vi "auto foil kinematics kl v4.1 08 01 2016.vi"() -> ()   [LabVIEW 2013]
uses:
  <vilib>/Utility/file.llb/Write To Spreadsheet File (DBL).vi
  <vilib>/Utility/file.llb/Write To Spreadsheet File (string).vi
  <vilib>/vision/NI_Vision_Development_Module.lvlib
panel:
  in  "X coordinate \nwithin gap\n(in pixels)":dbl=550.0
  in  "ON for 2 foil\nsegments":bool
  in  "Start frame":i32=1
  in  "ON to \nsimulate rod":bool
  in  "ON for pitch,\nOFF if NO pitch":bool=TRUE
  in  "Rod width (mm)":dbl=10.0
  out "Rotated/Mirrored image":T1(plugin-control)
  in  "Frame increment\nfor kinematics avi":i32=20
  in  "Flip along\nhorizontal line":bool
  in  "Flip along\nvertical line":bool
  in  "Save amps of\noscillation\nto txt file":bool
  in  "Save splines\nfor snapshot\ngeneration":bool
  in  "File path for snapshot splines (dialog if empty)":path=path "C:/Users/Lauder Lab/Desktop/snapshotstest.txt"
  in  "Number of\ncycles":i32=2
  in  "Foil chord (m)":dbl=0.18
  in  "File path for amplitudes of oscillation (dialog if empty)":path=path "C:/Users/Lauder Lab/Desktop/testcol.txt"
  in  "Increment for\nsaving extra\n splines":i32=20
  in  "File path for extra kinematics splines (dialog if empty)":path=path "C:/Users/Lauder Lab/Desktop/splinestest.txt"
  in  "For raw detected\nsurface:\nOn for mm,\nOff for pixels":bool
  in  "Save raw \ndetected\nsurface to\nspreadsheet":bool
  in  "File path for surfaces (dialog if empty)":path=path "C:/Users/Lauder Lab/Desktop/test.txt"
  in  "Save extra splines\n(at increment)\nto txt file":bool
  in  "Save an avi\nanimation":bool
  in  "File path for kinematics avi":path=path "C:/Users/Lauder Lab/Desktop/movie.avi"
  in  "Rotate\n90 deg (CCW)":bool
  in  "Rotate\n180 deg":bool
  in  "On for\ntest display":bool=TRUE
  in  "Number of frames\nto analyze":i32=1000
  out "surface":cluster{i32, "Rows":i32}[](graph)=[{0, "Rows"=0}, {1, "Rows"=0}, {2, "Rows"=0}, {3, "Rows"=0}, {4, "Rows"=0}, {5, "Rows"=0}, {6, "Rows"=0}, {7, "Rows"=0}, {8, "Rows"=0}, {9, "Rows"=0}, {10, "Rows"=0}, {11, "Rows"=0}, {12, "Rows"=0}, {13, "Rows"=0}, {14, "Rows"=0}, {15, "Rows"=0}, {16, "Rows"=0}, {17, "Rows"=0}, {18, "Rows"=0}, {19, "Rows"=0}, {20, "Rows"=0}, {21, "Rows"=0}, {22, "Rows"=0}, {23, "Rows"=0}, {24, "Rows"=0}, {25, "Rows"=0}, {26, "Rows"=0}, {27, "Rows"=0}, {28, "Rows"=0}, {29, "Rows"=0}, {30, "Rows"=0}, {31, "Rows"=0}, {32, "Rows"=0}, {33, "Rows"=0}, {34, "Rows"=0}, {35, "Rows"=0}, {36, "Rows"=0}, {37, "Rows"=0}, {38, "Rows"=0}, {39, "Rows"=0}, {40, "Rows"=0}, {41, "Rows"=0}, {42, "Rows"=0}, {43, "Rows"=0}, {44, "Rows"=0}, {45, "Rows"=0}, {46, "Rows"=0}, {47, "Rows"=0}, {48, "Rows"=0}, {49, "Rows"=0}, {50, "Rows"=0}, {51, "Rows"=0}, {52, "Rows"=0}, {53, "Rows"=0}, {54, "Rows"=0}, {55, "Rows"=0}, {56, "Rows"=0}, {57, "Rows"=0}, {58, "Rows"=0}, {59, "Rows"=0}, {60, "Rows"=0}, {61, "Rows"=0}, {62, "Rows"=0}, {63, "Rows"=0}, {64, "Rows"=0}, {65, "Rows"=0}, {66, "Rows"=0}, {67, "Rows"=0}, {68, "Rows"=0}, {69, "Rows"=0}, {70, "Rows"=0}, {71, "Rows"=0}, {72, "Rows"=0}, {73, "Rows"=0}, {74, "Rows"=0}, {75, "Rows"=0}, {76, "Rows"=0}, {77, "Rows"=0}, {78, "Rows"=0}, {79, "Rows"=0}, {80, "Rows"=0}, {81, "Rows"=0}, {82, "Rows"=0}, {83, "Rows"=0}, {84, "Rows"=0}, {85, "Rows"=0}, {86, "Rows"=0}, {87, "Rows"=0}, {88, "Rows"=0}, {89, "Rows"=0}, {90, "Rows"=0}, {91, "Rows"=0}, {92, "Rows"=0}, {93, "Rows"=0}, {94, "Rows"=0}, {95, "Rows"=0}, {96, "Rows"=0}, {97, "Rows"=0}, {98, "Rows"=0}, {99, "Rows"=0}, {100, "Rows"=0}, {101, "Rows"=0}, {102, "Rows"=0}, {103, "Rows"=0}, {104, "Rows"=0}, {105, "Rows"=0}, {106, "Rows"=0}, {107, "Rows"=0}, {108, "Rows"=0}, {109, "Rows"=0}, {110, "Rows"=0}, {111, "Rows"=0}, {112, "Rows"=0}, {113, "Rows"=0}, {114, "Rows"=0}, {115, "Rows"=0}, {116, "Rows"=0}, {117, "Rows"=0}, {118, "Rows"=0}, {119, "Rows"=0}, {120, "Rows"=0}, {121, "Rows"=0}, {122, "Rows"=0}, {123, "Rows"=0}, {124, "Rows"=0}, {125, "Rows"=0}, {126, "Rows"=0}, {127, "Rows"=0}, {128, "Rows"=0}, {129, "Rows"=0}, {130, "Rows"=0}, {131, "Rows"=0}, {132, "Rows"=0}, {133, "Rows"=0}, {134, "Rows"=0}, {135, "Rows"=0}, {136, "Rows"=0}, {137, "Rows"=0}, {138, "Rows"=0}, {139, "Rows"=0}, {140, "Rows"=0}, {141, "Rows"=0}, {142, "Rows"=0}, {143, "Rows"=0}, {144, "Rows"=0}, {145, "Rows"=0}, {146, "Rows"=0}, {147, "Rows"=0}, {148, "Rows"=0}, {149, "Rows"=0}, {150, "Rows"=0}, {151, "Rows"=0}, {152, "Rows"=0}, {153, "Rows"=0}, {154, "Rows"=0}, {155, "Rows"=0}, {156, "Rows"=0}, {157, "Rows"=0}, {158, "Rows"=0}, {159, "Rows"=0}, {160, "Rows"=0}, {161, "Rows"=0}, {162, "Rows"=0}, {163, "Rows"=0}, {164, "Rows"=0}, {165, "Rows"=0}, {166, "Rows"=0}, {167, "Rows"=0}, {168, "Rows"=0}, {169, "Rows"=0}, {170, "Rows"=0}, {171, "Rows"=0}, {172, "Rows"=0}, {173, "Rows"=0}, {174, "Rows"=0}, {175, "Rows"=0}, {176, "Rows"=0}, {177, "Rows"=0}, {178, "Rows"=0}, {179, "Rows"=0}, {180, "Rows"=0}, {181, "Rows"=0}, {182, "Rows"=0}, {183, "Rows"=0}, {184, "Rows"=0}, {185, "Rows"=0}, {186, "Rows"=0}, {187, "Rows"=0}, {188, "Rows"=0}, {189, "Rows"=0}, {190, "Rows"=0}, {191, "Rows"=0}, {192, "Rows"=0}, {193, "Rows"=0}, {194, "Rows"=0}, {195, "Rows"=0}, {196, "Rows"=0}, {197, "Rows"=0}, {198, "Rows"=0}, {199, "Rows"=0}, {200, "Rows"=0}, {201, "Rows"=0}, {202, "Rows"=0}, {203, "Rows"=0}, {204, "Rows"=0}, {205, "Rows"=0}, {206, "Rows"=0}, {207, "Rows"=0}, {208, "Rows"=0}, {209, "Rows"=0}, {210, "Rows"=0}, {211, "Rows"=0}, {212, "Rows"=0}, {213, "Rows"=0}, {214, "Rows"=0}, {215, "Rows"=0}, {216, "Rows"=0}, {217, "Rows"=0}, {218, "Rows"=0}, {219, "Rows"=0}, {220, "Rows"=0}, {221, "Rows"=0}, {222, "Rows"=0}, {223, "Rows"=0}, {224, "Rows"=0}, {225, "Rows"=582}, {226, "Rows"=582}, {227, "Rows"=581}, {228, "Rows"=580}, {229, "Rows"=579}, {230, "Rows"=579}, {231, "Rows"=579}, {232, "Rows"=579}, {233, "Rows"=579}, {234, "Rows"=579}, {235, "Rows"=579}, {236, "Rows"=579}, {237, "Rows"=579}, {238, "Rows"=579}, {239, "Rows"=579}, {240, "Rows"=579}, {241, "Rows"=579}, {242, "Rows"=578}, {243, "Rows"=578}, {244, "Rows"=578}, {245, "Rows"=578}, {246, "Rows"=578}, {247, "Rows"=578}, {248, "Rows"=578}, {249, "Rows"=578}, {250, "Rows"=578}, {251, "Rows"=578}, {252, "Rows"=578}, {253, "Rows"=578}, {254, "Rows"=578}, {255, "Rows"=578}, {256, "Rows"=578}, {257, "Rows"=578}, {258, "Rows"=577}, {259, "Rows"=577}, {260, "Rows"=577}, {261, "Rows"=577}, {262, "Rows"=577}, {263, "Rows"=577}, {264, "Rows"=577}, {265, "Rows"=577}, {266, "Rows"=577}, {267, "Rows"=577}, {268, "Rows"=577}, {269, "Rows"=577}, {270, "Rows"=577}, {271, "Rows"=577}, {272, "Rows"=577}, {273, "Rows"=577}, {274, "Rows"=577}, {275, "Rows"=577}, {276, "Rows"=576}, {277, "Rows"=576}, {278, "Rows"=576}, {279, "Rows"=576}, {280, "Rows"=576}, {281, "Rows"=576}, {282, "Rows"=576}, {283, "Rows"=576}, {284, "Rows"=576}, {285, "Rows"=576}, {286, "Rows"=576}, {287, "Rows"=576}, {288, "Rows"=576}, {289, "Rows"=576}, {290, "Rows"=576}, {291, "Rows"=576}, {292, "Rows"=576}, {293, "Rows"=575}, {294, "Rows"=575}, {295, "Rows"=575}, {296, "Rows"=575}, {297, "Rows"=575}, {298, "Rows"=575}, {299, "Rows"=575}, {300, "Rows"=575}, {301, "Rows"=575}, {302, "Rows"=574}, {303, "Rows"=574}, {304, "Rows"=574}, {305, "Rows"=574}, {306, "Rows"=574}, {307, "Rows"=574}, {308, "Rows"=574}, {309, "Rows"=574}, {310, "Rows"=574}, {311, "Rows"=574}, {312, "Rows"=574}, {313, "Rows"=574}, {314, "Rows"=573}, {315, "Rows"=573}, {316, "Rows"=573}, {317, "Rows"=573}, {318, "Rows"=573}, {319, "Rows"=573}, {320, "Rows"=573}, {321, "Rows"=573}, {322, "Rows"=573}, {323, "Rows"=573}, {324, "Rows"=572}, {325, "Rows"=572}, {326, "Rows"=572}, {327, "Rows"=572}, {328, "Rows"=572}, {329, "Rows"=572}, {330, "Rows"=572}, {331, "Rows"=572}, {332, "Rows"=571}, {333, "Rows"=572}, {334, "Rows"=571}, {335, "Rows"=571}, {336, "Rows"=571}, {337, "Rows"=571}, {338, "Rows"=570}, {339, "Rows"=571}, {340, "Rows"=571}, {341, "Rows"=570}, {342, "Rows"=570}, {343, "Rows"=570}, {344, "Rows"=570}, {345, "Rows"=570}, {346, "Rows"=570}, {347, "Rows"=570}, {348, "Rows"=569}, {349, "Rows"=569}, {350, "Rows"=569}, {351, "Rows"=569}, {352, "Rows"=569}, {353, "Rows"=569}, {354, "Rows"=569}, {355, "Rows"=569}, {356, "Rows"=568}, {357, "Rows"=568}, {358, "Rows"=568}, {359, "Rows"=568}, {360, "Rows"=568}, {361, "Rows"=568}, {362, "Rows"=567}, {363, "Rows"=567}, {364, "Rows"=567}, {365, "Rows"=567}, {366, "Rows"=567}, {367, "Rows"=566}, {368, "Rows"=566}, {369, "Rows"=566}, {370, "Rows"=566}, {371, "Rows"=566}, {372, "Rows"=566}, {373, "Rows"=565}, {374, "Rows"=565}, {375, "Rows"=565}, {376, "Rows"=565}, {377, "Rows"=565}, {378, "Rows"=565}, {379, "Rows"=564}, {380, "Rows"=564}, {381, "Rows"=564}, {382, "Rows"=564}, {383, "Rows"=564}, {384, "Rows"=564}, {385, "Rows"=564}, {386, "Rows"=563}, {387, "Rows"=563}, {388, "Rows"=563}, {389, "Rows"=563}, {390, "Rows"=562}, {391, "Rows"=562}, {392, "Rows"=562}, {393, "Rows"=562}, {394, "Rows"=562}, {395, "Rows"=562}, {396, "Rows"=562}, {397, "Rows"=561}, {398, "Rows"=561}, {399, "Rows"=561}, {400, "Rows"=561}, {401, "Rows"=561}, {402, "Rows"=560}, {403, "Rows"=560}, {404, "Rows"=560}, {405, "Rows"=560}, {406, "Rows"=560}, {407, "Rows"=560}, {408, "Rows"=560}, {409, "Rows"=559}, {410, "Rows"=559}, {411, "Rows"=559}, {412, "Rows"=559}, {413, "Rows"=558}, {414, "Rows"=558}, {415, "Rows"=558}, {416, "Rows"=558}, {417, "Rows"=558}, {418, "Rows"=557}, {419, "Rows"=557}, {420, "Rows"=557}, {421, "Rows"=557}, {422, "Rows"=557}, {423, "Rows"=557}, {424, "Rows"=556}, {425, "Rows"=556}, {426, "Rows"=556}, {427, "Rows"=556}, {428, "Rows"=556}, {429, "Rows"=555}, {430, "Rows"=555}, {431, "Rows"=555}, {432, "Rows"=555}, {433, "Rows"=554}, {434, "Rows"=554}, {435, "Rows"=554}, {436, "Rows"=554}, {437, "Rows"=554}, {438, "Rows"=554}, {439, "Rows"=553}, {440, "Rows"=553}, {441, "Rows"=553}, {442, "Rows"=553}, {443, "Rows"=553}, {444, "Rows"=553}, {445, "Rows"=552}, {446, "Rows"=552}, {447, "Rows"=552}, {448, "Rows"=552}, {449, "Rows"=552}, {450, "Rows"=551}, {451, "Rows"=551}, {452, "Rows"=551}, {453, "Rows"=551}, {454, "Rows"=550}, {455, "Rows"=550}, {456, "Rows"=550}, {457, "Rows"=550}, {458, "Rows"=550}, {459, "Rows"=549}, {460, "Rows"=549}, {461, "Rows"=549}, {462, "Rows"=549}, {463, "Rows"=549}, {464, "Rows"=548}, {465, "Rows"=548}, {466, "Rows"=548}, {467, "Rows"=548}, {468, "Rows"=548}, {469, "Rows"=548}, {470, "Rows"=547}, {471, "Rows"=547}, {472, "Rows"=547}, {473, "Rows"=547}, {474, "Rows"=547}, {475, "Rows"=546}, {476, "Rows"=546}, {477, "Rows"=546}, {478, "Rows"=546}, {479, "Rows"=546}, {480, "Rows"=546}, {481, "Rows"=546}, {482, "Rows"=545}, {483, "Rows"=545}, {484, "Rows"=545}, {485, "Rows"=545}, {486, "Rows"=544}, {487, "Rows"=544}, {488, "Rows"=544}, {489, "Rows"=544}, {490, "Rows"=544}, {491, "Rows"=541}, {492, "Rows"=541}, {493, "Rows"=543}, {494, "Rows"=543}, {495, "Rows"=542}, {496, "Rows"=542}, {497, "Rows"=542}, {498, "Rows"=542}, {499, "Rows"=541}, {500, "Rows"=541}, {501, "Rows"=541}, {502, "Rows"=541}, {503, "Rows"=541}, {504, "Rows"=541}, {505, "Rows"=540}, {506, "Rows"=540}, {507, "Rows"=540}, {508, "Rows"=540}, {509, "Rows"=540}, {510, "Rows"=539}, {511, "Rows"=539}, {512, "Rows"=539}, {513, "Rows"=539}, {514, "Rows"=539}, {515, "Rows"=538}, {516, "Rows"=538}, {517, "Rows"=538}, {518, "Rows"=537}, {519, "Rows"=537}, {520, "Rows"=537}, {521, "Rows"=537}, {522, "Rows"=537}, {523, "Rows"=536}, {524, "Rows"=536}, {525, "Rows"=536}, {526, "Rows"=536}, {527, "Rows"=536}, {528, "Rows"=535}, {529, "Rows"=535}, {530, "Rows"=535}, {531, "Rows"=535}, {532, "Rows"=535}, {533, "Rows"=534}, {534, "Rows"=534}, {535, "Rows"=534}, {536, "Rows"=534}, {537, "Rows"=534}, {538, "Rows"=533}, {539, "Rows"=533}, {540, "Rows"=533}, {541, "Rows"=533}, {542, "Rows"=533}, {543, "Rows"=532}, {544, "Rows"=532}, {545, "Rows"=532}, {546, "Rows"=532}, {547, "Rows"=532}, {548, "Rows"=531}, {549, "Rows"=531}, {550, "Rows"=531}, {551, "Rows"=531}, {552, "Rows"=531}, {553, "Rows"=530}, {554, "Rows"=530}, {555, "Rows"=530}, {556, "Rows"=530}, {557, "Rows"=530}, {558, "Rows"=530}, {559, "Rows"=529}, {560, "Rows"=529}, {561, "Rows"=529}, {562, "Rows"=529}, {563, "Rows"=528}, {564, "Rows"=528}, {565, "Rows"=528}, {566, "Rows"=528}, {567, "Rows"=527}, {568, "Rows"=527}, {569, "Rows"=527}, {570, "Rows"=527}, {571, "Rows"=526}, {572, "Rows"=526}, {573, "Rows"=526}, {574, "Rows"=526}, {575, "Rows"=526}, {576, "Rows"=526}, {577, "Rows"=525}, {578, "Rows"=525}, {579, "Rows"=525}, {580, "Rows"=524}, {581, "Rows"=524}, {582, "Rows"=524}, {583, "Rows"=524}, {584, "Rows"=524}, {585, "Rows"=524}, {586, "Rows"=524}, {587, "Rows"=523}, {588, "Rows"=523}, {589, "Rows"=523}, {590, "Rows"=523}, {591, "Rows"=522}, {592, "Rows"=522}, {593, "Rows"=522}, {594, "Rows"=522}, {595, "Rows"=520}, {596, "Rows"=521}, {597, "Rows"=521}, {598, "Rows"=521}, {599, "Rows"=520}, {600, "Rows"=520}, {601, "Rows"=520}, {602, "Rows"=520}, {603, "Rows"=519}, {604, "Rows"=519}, {605, "Rows"=519}, {606, "Rows"=519}, {607, "Rows"=518}, {608, "Rows"=518}, {609, "Rows"=517}, {610, "Rows"=517}, {611, "Rows"=517}, {612, "Rows"=516}, {613, "Rows"=516}, {614, "Rows"=516}, {615, "Rows"=516}, {616, "Rows"=516}, {617, "Rows"=516}, {618, "Rows"=516}, {619, "Rows"=516}, {620, "Rows"=516}, {621, "Rows"=516}, {622, "Rows"=516}, {623, "Rows"=516}, {624, "Rows"=515}, {625, "Rows"=514}, {626, "Rows"=513}, {627, "Rows"=513}, {628, "Rows"=513}, {629, "Rows"=513}, {630, "Rows"=513}, {631, "Rows"=512}, {632, "Rows"=512}, {633, "Rows"=511}, {634, "Rows"=511}, {635, "Rows"=511}, {636, "Rows"=511}, {637, "Rows"=511}, {638, "Rows"=510}, {639, "Rows"=510}, {640, "Rows"=509}, {641, "Rows"=508}, {642, "Rows"=508}, {643, "Rows"=507}, {644, "Rows"=507}, {645, "Rows"=507}, {646, "Rows"=506}, {647, "Rows"=506}, {648, "Rows"=505}, {649, "Rows"=505}, {650, "Rows"=504}, {651, "Rows"=504}, {652, "Rows"=504}, {653, "Rows"=503}, {654, "Rows"=502}, {655, "Rows"=501}, {656, "Rows"=501}, {657, "Rows"=501}, {658, "Rows"=500}, {659, "Rows"=499}, {660, "Rows"=498}, {661, "Rows"=498}, {662, "Rows"=498}, {663, "Rows"=498}, {664, "Rows"=497}, {665, "Rows"=496}, {666, "Rows"=496}, {667, "Rows"=495}, {668, "Rows"=494}, {669, "Rows"=494}, {670, "Rows"=493}, {671, "Rows"=493}, {672, "Rows"=492}, {673, "Rows"=491}, {674, "Rows"=491}, {675, "Rows"=490}, {676, "Rows"=489}, {677, "Rows"=489}, {678, "Rows"=488}, {679, "Rows"=488}, {680, "Rows"=487}, {681, "Rows"=486}, {682, "Rows"=486}, {683, "Rows"=485}, {684, "Rows"=484}, {685, "Rows"=483}, {686, "Rows"=483}, {687, "Rows"=482}, {688, "Rows"=481}, {689, "Rows"=480}, {690, "Rows"=479}, {691, "Rows"=479}, {692, "Rows"=478}, {693, "Rows"=478}, {694, "Rows"=477}, {695, "Rows"=476}, {696, "Rows"=476}, {697, "Rows"=475}, {698, "Rows"=474}, {699, "Rows"=473}, {700, "Rows"=472}, {701, "Rows"=472}, {702, "Rows"=471}, {703, "Rows"=470}, {704, "Rows"=470}, {705, "Rows"=469}, {706, "Rows"=468}, {707, "Rows"=467}, {708, "Rows"=467}, {709, "Rows"=466}, {710, "Rows"=464}, {711, "Rows"=463}, {712, "Rows"=463}, {713, "Rows"=463}, {714, "Rows"=462}, {715, "Rows"=461}, {716, "Rows"=460}, {717, "Rows"=459}, {718, "Rows"=458}, {719, "Rows"=458}, {720, "Rows"=457}, {721, "Rows"=456}, {722, "Rows"=455}, {723, "Rows"=455}, {724, "Rows"=454}, {725, "Rows"=453}, {726, "Rows"=452}, {727, "Rows"=451}, {728, "Rows"=450}, {729, "Rows"=450}, {730, "Rows"=449}, {731, "Rows"=448}, {732, "Rows"=447}, {733, "Rows"=447}, {734, "Rows"=446}, {735, "Rows"=445}, {736, "Rows"=444}, {737, "Rows"=443}, {738, "Rows"=442}, {739, "Rows"=441}, {740, "Rows"=440}, {741, "Rows"=439}, {742, "Rows"=438}, {743, "Rows"=438}, {744, "Rows"=437}, {745, "Rows"=436}, {746, "Rows"=436}, {747, "Rows"=435}, {748, "Rows"=434}, {749, "Rows"=433}, {750, "Rows"=432}, {751, "Rows"=432}, {752, "Rows"=431}, {753, "Rows"=430}, {754, "Rows"=429}, {755, "Rows"=428}, {756, "Rows"=427}, {757, "Rows"=426}, {758, "Rows"=425}, {759, "Rows"=425}, {760, "Rows"=424}, {761, "Rows"=423}, {762, "Rows"=422}, {763, "Rows"=421}, {764, "Rows"=420}, {765, "Rows"=420}, {766, "Rows"=419}, {767, "Rows"=418}, {768, "Rows"=417}, {769, "Rows"=416}, {770, "Rows"=415}, {771, "Rows"=415}, {772, "Rows"=414}, {773, "Rows"=413}, {774, "Rows"=412}, {775, "Rows"=411}, {776, "Rows"=410}, {777, "Rows"=410}, {778, "Rows"=409}, {779, "Rows"=408}, {780, "Rows"=407}, {781, "Rows"=406}, {782, "Rows"=405}, {783, "Rows"=404}, {784, "Rows"=403}, {785, "Rows"=402}, {786, "Rows"=401}, {787, "Rows"=401}, {788, "Rows"=400}, {789, "Rows"=399}, {790, "Rows"=398}, {791, "Rows"=398}, {792, "Rows"=398}, {793, "Rows"=399}, {794, "Rows"=0}, {795, "Rows"=0}, {796, "Rows"=0}, {797, "Rows"=0}, {798, "Rows"=0}, {799, "Rows"=0}, {800, "Rows"=0}, {801, "Rows"=0}, {802, "Rows"=0}, {803, "Rows"=0}, {804, "Rows"=0}, {805, "Rows"=0}, {806, "Rows"=0}, {807, "Rows"=0}, {808, "Rows"=0}, {809, "Rows"=0}, {810, "Rows"=0}, {811, "Rows"=0}, {812, "Rows"=0}, {813, "Rows"=0}, {814, "Rows"=0}, {815, "Rows"=0}, {816, "Rows"=0}, {817, "Rows"=0}, {818, "Rows"=0}, {819, "Rows"=0}, {820, "Rows"=0}, {821, "Rows"=0}, {822, "Rows"=0}, {823, "Rows"=0}, {824, "Rows"=0}, {825, "Rows"=0}, {826, "Rows"=0}, {827, "Rows"=0}, {828, "Rows"=0}, {829, "Rows"=0}, {830, "Rows"=0}, {831, "Rows"=0}, {832, "Rows"=0}, {833, "Rows"=0}, {834, "Rows"=0}, {835, "Rows"=0}, {836, "Rows"=0}, {837, "Rows"=0}, {838, "Rows"=0}, {839, "Rows"=0}, {840, "Rows"=0}, {841, "Rows"=0}, {842, "Rows"=0}, {843, "Rows"=0}, {844, "Rows"=0}, {845, "Rows"=0}, {846, "Rows"=0}, {847, "Rows"=0}, {848, "Rows"=0}, {849, "Rows"=0}, {850, "Rows"=0}, {851, "Rows"=0}, {852, "Rows"=0}, {853, "Rows"=0}, {854, "Rows"=0}, {855, "Rows"=0}, {856, "Rows"=0}, {857, "Rows"=0}, {858, "Rows"=0}, {859, "Rows"=0}, {860, "Rows"=0}, {861, "Rows"=0}, {862, "Rows"=0}, {863, "Rows"=0}, {864, "Rows"=0}, {865, "Rows"=0}, {866, "Rows"=0}, {867, "Rows"=0}, {868, "Rows"=0}, {869, "Rows"=0}, {870, "Rows"=0}, {871, "Rows"=0}, {872, "Rows"=0}, {873, "Rows"=0}, {874, "Rows"=0}, {875, "Rows"=0}, {876, "Rows"=0}, {877, "Rows"=0}, {878, "Rows"=0}, {879, "Rows"=0}, {880, "Rows"=0}, {881, "Rows"=0}, {882, "Rows"=0}, {883, "Rows"=0}, {884, "Rows"=0}, {885, "Rows"=0}, {886, "Rows"=0}, {887, "Rows"=0}, {888, "Rows"=0}, {889, "Rows"=0}, {890, "Rows"=0}, {891, "Rows"=0}, {892, "Rows"=0}, {893, "Rows"=0}, {894, "Rows"=0}, {895, "Rows"=0}, {896, "Rows"=0}, {897, "Rows"=0}, {898, "Rows"=0}, {899, "Rows"=0}, {900, "Rows"=0}, {901, "Rows"=0}, {902, "Rows"=0}, {903, "Rows"=0}, {904, "Rows"=0}, {905, "Rows"=0}, {906, "Rows"=0}, {907, "Rows"=0}, {908, "Rows"=0}, {909, "Rows"=0}, {910, "Rows"=0}, {911, "Rows"=0}, {912, "Rows"=0}, {913, "Rows"=0}, {914, "Rows"=0}, {915, "Rows"=0}, {916, "Rows"=0}, {917, "Rows"=0}, {918, "Rows"=0}, {919, "Rows"=0}, {920, "Rows"=0}, {921, "Rows"=0}, {922, "Rows"=0}, {923, "Rows"=0}, {924, "Rows"=0}, {925, "Rows"=0}, {926, "Rows"=0}, {927, "Rows"=0}, {928, "Rows"=0}, {929, "Rows"=0}, {930, "Rows"=0}, {931, "Rows"=0}, {932, "Rows"=0}, {933, "Rows"=0}, {934, "Rows"=0}, {935, "Rows"=0}, {936, "Rows"=0}, {937, "Rows"=0}, {938, "Rows"=0}, {939, "Rows"=0}, {940, "Rows"=0}, {941, "Rows"=0}, {942, "Rows"=0}, {943, "Rows"=0}, {944, "Rows"=0}, {945, "Rows"=0}, {946, "Rows"=0}, {947, "Rows"=0}, {948, "Rows"=0}, {949, "Rows"=0}, {950, "Rows"=0}, {951, "Rows"=0}, {952, "Rows"=0}, {953, "Rows"=0}, {954, "Rows"=0}, {955, "Rows"=0}, {956, "Rows"=0}, {957, "Rows"=0}, {958, "Rows"=0}, {959, "Rows"=0}, {960, "Rows"=0}, {961, "Rows"=0}, {962, "Rows"=0}, {963, "Rows"=0}, {964, "Rows"=0}, {965, "Rows"=0}, {966, "Rows"=0}, {967, "Rows"=0}, {968, "Rows"=0}, {969, "Rows"=0}, {970, "Rows"=0}, {971, "Rows"=0}, {972, "Rows"=0}, {973, "Rows"=0}, {974, "Rows"=0}, {975, "Rows"=0}, {976, "Rows"=0}, {977, "Rows"=0}, {978, "Rows"=0}, {979, "Rows"=0}, {980, "Rows"=0}, {981, "Rows"=0}, {982, "Rows"=0}, {983, "Rows"=0}, {984, "Rows"=0}, {985, "Rows"=0}, {986, "Rows"=0}, {987, "Rows"=0}, {988, "Rows"=0}, {989, "Rows"=0}, {990, "Rows"=0}, {991, "Rows"=0}, {992, "Rows"=0}, {993, "Rows"=0}, {994, "Rows"=0}, {995, "Rows"=0}, {996, "Rows"=0}, {997, "Rows"=0}, {998, "Rows"=0}, {999, "Rows"=0}, {1000, "Rows"=0}, {1001, "Rows"=0}, {1002, "Rows"=0}, {1003, "Rows"=0}, {1004, "Rows"=0}, {1005, "Rows"=0}, {1006, "Rows"=0}, {1007, "Rows"=0}, {1008, "Rows"=0}, {1009, "Rows"=0}, {1010, "Rows"=0}, {1011, "Rows"=0}, {1012, "Rows"=0}, {1013, "Rows"=0}, {1014, "Rows"=0}, {1015, "Rows"=0}, {1016, "Rows"=0}, {1017, "Rows"=0}, {1018, "Rows"=0}, {1019, "Rows"=0}, {1020, "Rows"=0}, {1021, "Rows"=0}, {1022, "Rows"=0}, {1023, "Rows"=0}]
  in  "use max\npixel for \nsurface":bool=TRUE
  in  "surface finder settings":T2={"pixel column start index"=220, "pixel column end index"=800, "analyze all\nimage\ncolumns"=FALSE, "surface pixel offset"=0, "lowest pix intensity\nfor surface id"=100, "intensity step\nsize for search"=10, "maximum expected\nparticle width"=3, "slope of intensity\nfor surface peak id"=0.5, "no body\npresent"=FALSE, "edge position\nhigh limit"=1007, "DaVis pixel\nscale factor\n(mm/pixel)"=0.304521}
  out "Image":T1(plugin-control)
  out "Y Resolution":i32=1024
  out "X Resolution":i32=1024
  in  "Selection Values":T4(array[cluster])=[{"Measurement Parameter"=35, "Range Lower Value"=200.0, "Range Upper Value"=10000.0, "Range"=FALSE, "Measurement Type"=FALSE}] {"Measurement Parameter" items=["Center of Mass X", "Center of Mass Y", "First Pixel X", "First Pixel Y", "Bounding Rect Left", "Bounding Rect Top", "Bounding Rect Right", "Bounding Rect Bottom", "Max Feret Diameter Start X", "Max Feret Diameter Start Y", "Max Feret Diameter End X", "Max Feret Diameter End Y", "Max Horiz. Segment Length Left", "Max Horiz. Segment Length Right", "Max Horiz. Segment Length Row", "-", "Bounding Rect Width", "Bounding Rect Height", "Bounding Rect Diagonal", "Perimeter", "Convex Hull Perimeter", "Holes' Perimeter", "Max Feret Diameter", "Equivalent Ellipse Major Axis", "Equivalent Ellipse Minor Axis", "Equivalent Ellipse Minor Axis (Feret)", "Equivalent Rect Long Side", "Equivalent Rect Short Side", "Equivalent Rect Diagonal", "Equivalent Rect Short Side (Feret)", "Average Horiz. Segment Length", "Average Vert. Segment Length", "Hydraulic Radius", "Waddel Disk Diameter", "-", "Area", "Holes' Area", "Particle & Holes' Area", "Convex Hull Area", "Image Area", "-", "Number of Holes", "Number of Horiz. Segments", "Number of Vert. Segments", "-", "Orientation", "Max Feret Diameter Orientation", "-", "% Area/Image Area", "% Area/(Particle & Holes' Area)", "Ratio of Equivalent Ellipse Axes", "Ratio of Equivalent Rect Sides", "-", "Elongation Factor", "Compactness Factor", "Heywood Circularity Factor", "Type Factor", "-", "Sum X", "Sum Y", "Sum XX", "Sum XY", "Sum YY", "Sum XXX", "Sum XXY", "Sum XYY", "Sum YYY", "-", "Moment of Inertia XX", "Moment of Inertia XY", "Moment of Inertia YY", "Moment of Inertia XXX", "Moment of Inertia XXY", "Moment of Inertia XYY", "Moment of Inertia YYY", "Norm. Moment of Inertia XX", "Norm. Moment of Inertia XY", "Norm. Moment of Inertia YY", "Norm. Moment of Inertia XXX", "Norm. Moment of Inertia XXY", "Norm. Moment of Inertia XYY", "Norm. Moment of Inertia YYY", "Hu Moment 1", "Hu Moment 2", "Hu Moment 3", "Hu Moment 4", "Hu Moment 5", "Hu Moment 6", "Hu Moment 7"]; "Range Lower Value" format="%.2f"; "Range Upper Value" format="%.2f"}
  in  "Range":cluster{"Lower value":sgl, "Upper value":sgl}={"Lower value"=180.0, "Upper value"=255.0} {"Upper value" format="%.2f"; "Lower value" format="%.2f"}
  out "current\nimage number":i32=22
  in  "Foil AVI file to load":path=path "G:/Oct3.foiltest.2013_paint/Glow.down.laserjustabove2.avi"
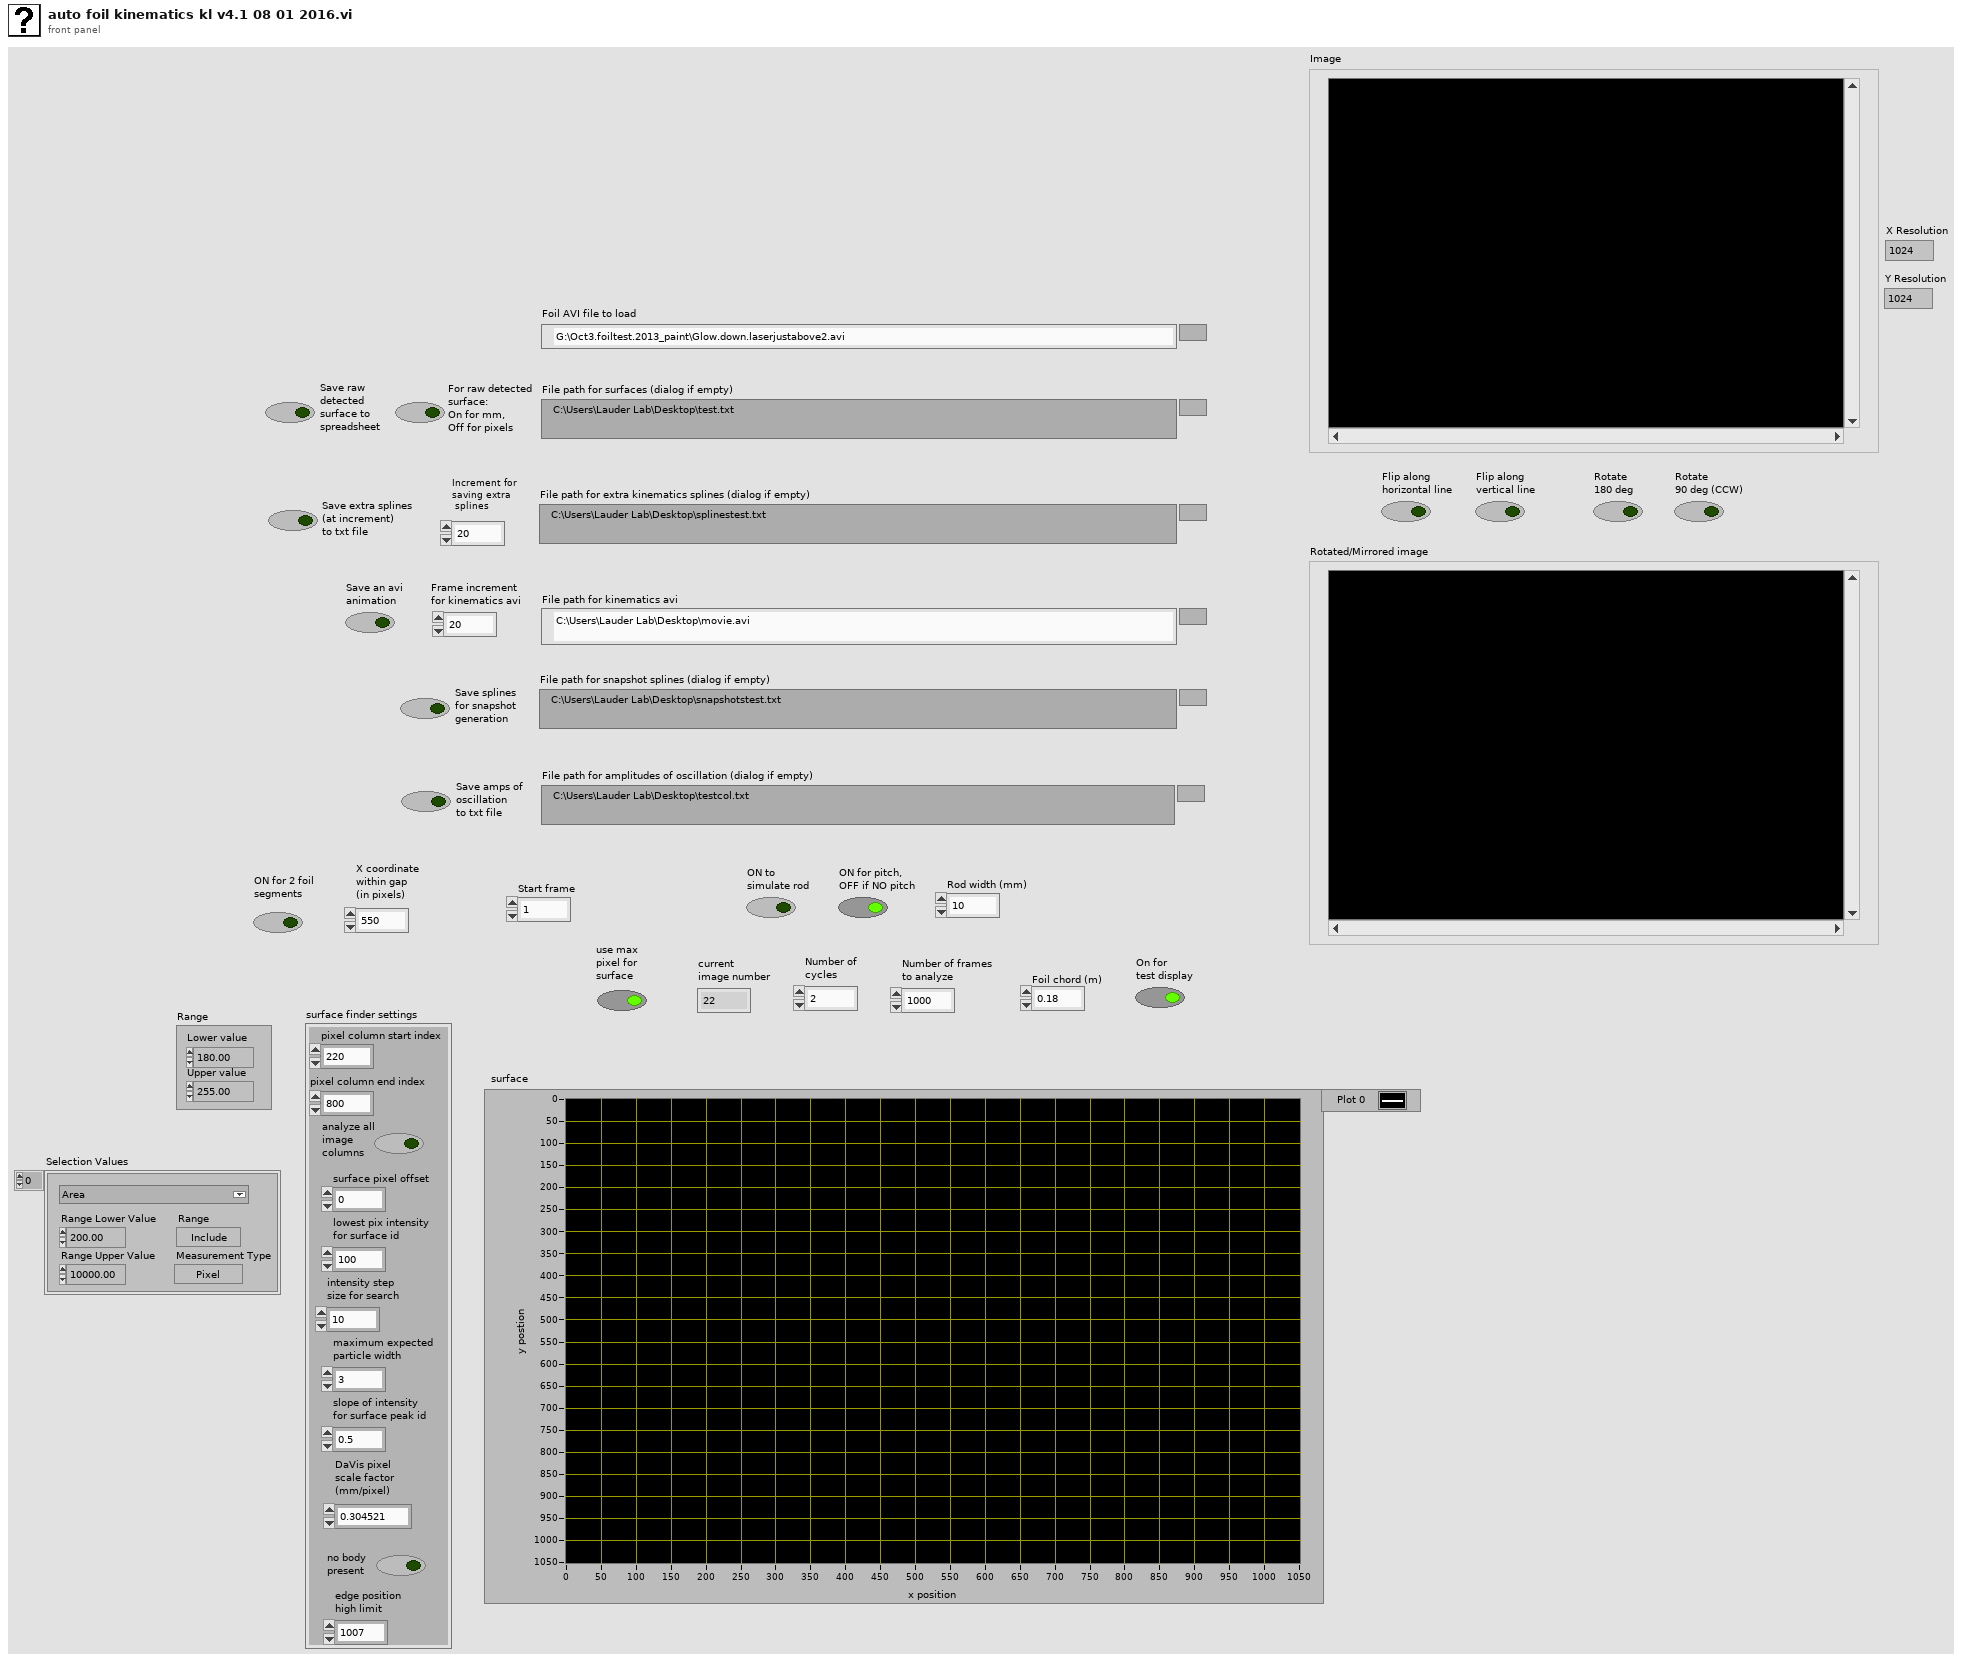
[diagram p1: front panel]
types:
  T1 = typedef "IMAQ Image.ctl" = refnum<image>
  T2 = cluster{"pixel column start index":i32, "pixel column end index":i32, "analyze all\nimage\ncolumns":bool, "surface pixel offset":i32, "lowest pix intensity\nfor surface id":i32, "intensity step\nsize for search":i32, "maximum expected\nparticle width":i32, "slope of intensity\nfor surface peak id":dbl, "no body\npresent":bool, "edge position\nhigh limit":i32, "DaVis pixel\nscale factor\n(mm/pixel)":dbl}
  T3 = typedef "Particle Parameters" = i32
  T4 = cluster{"Measurement Parameter":T3, "Range Lower Value":dbl, "Range Upper Value":dbl, "Range":bool, "Measurement Type":bool}[]
  T5 = enum32{"Gray", "Binary", "Gradient", "Rainbow", "Temperature"}
  T6 = typedef "Image Type" = u32
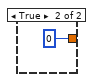
[diagram p3: hidden frame]
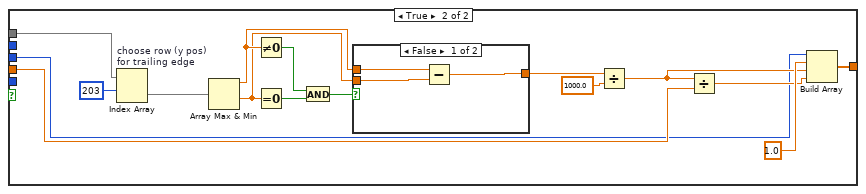
[diagram p4: hidden frame]
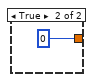
[diagram p5: hidden frame]
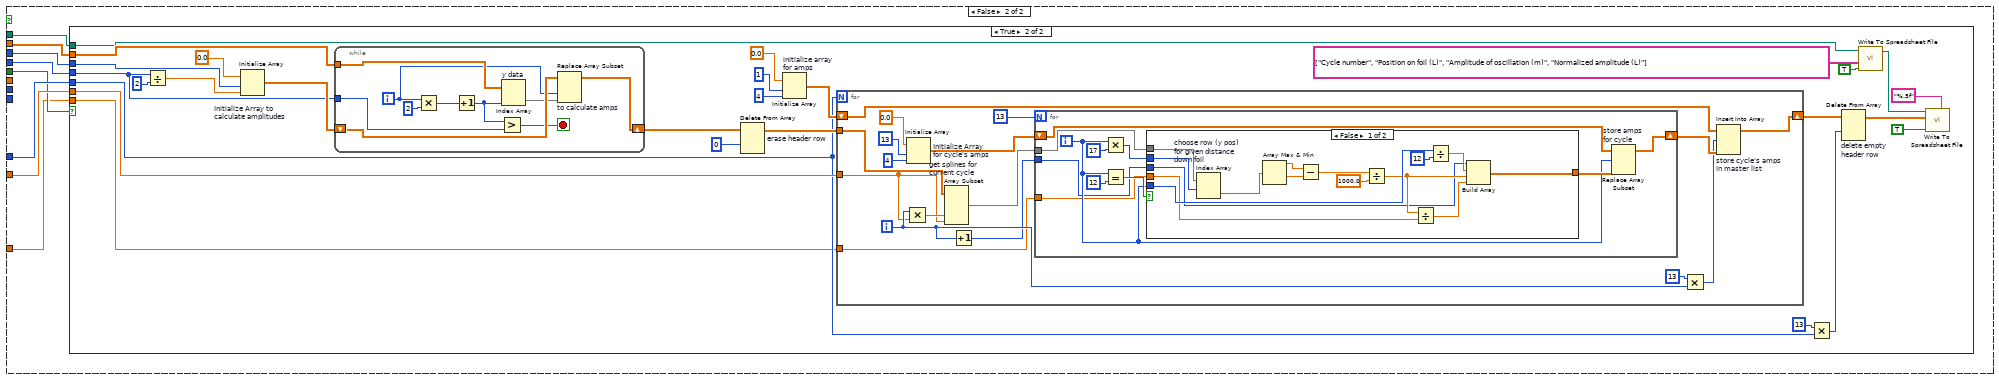
[diagram p6: hidden frame]
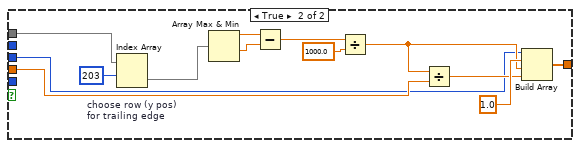
[diagram p8: hidden frame]
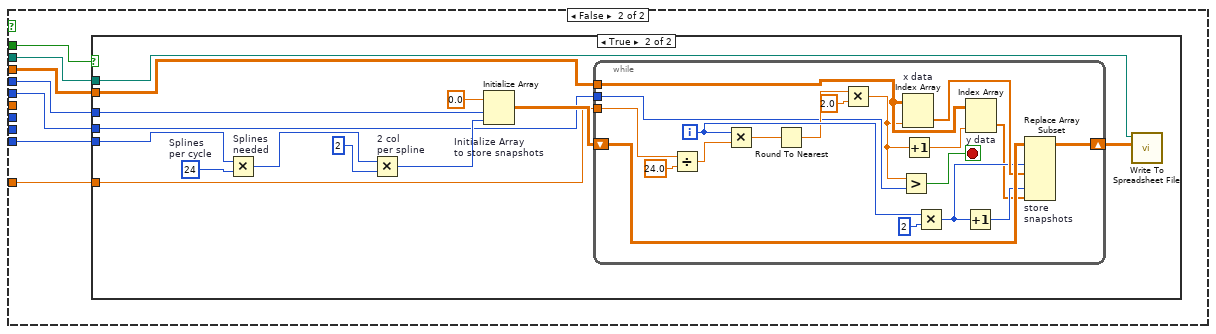
[diagram p10: hidden frame]
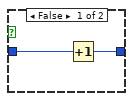
[diagram p14: hidden frame]
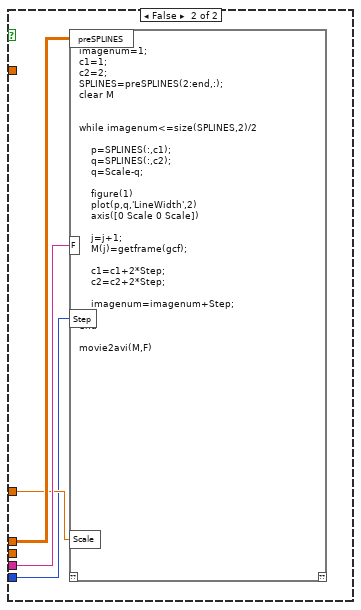
[diagram p16: hidden frame]
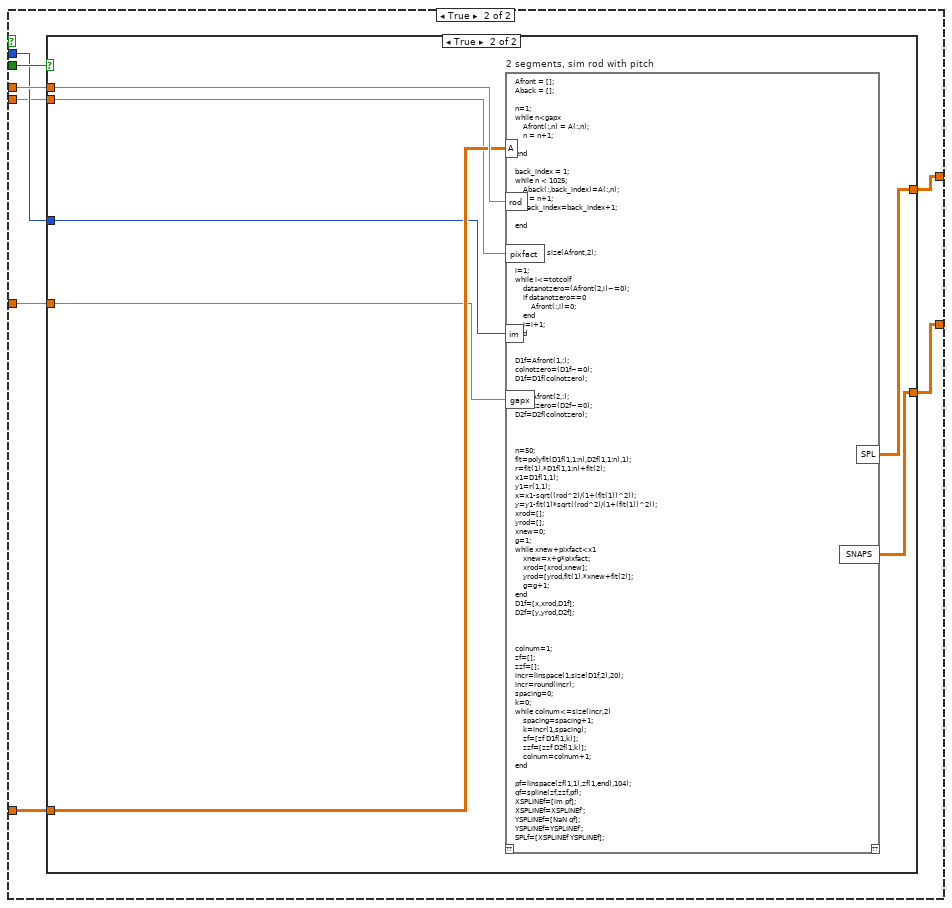
[diagram p18: hidden frame]
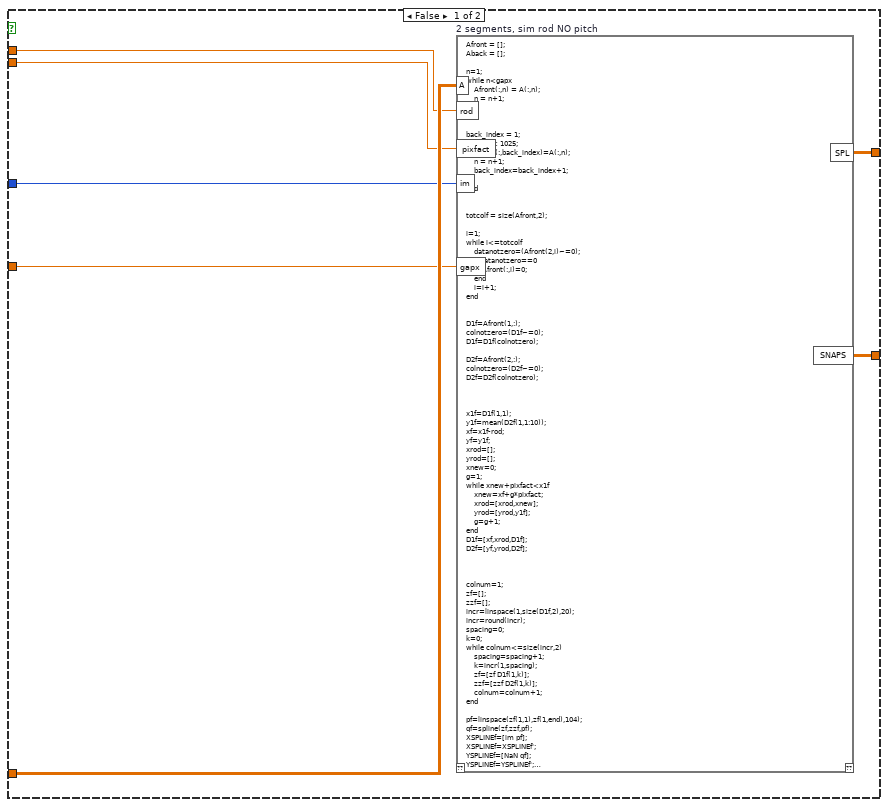
[diagram p19: hidden frame]
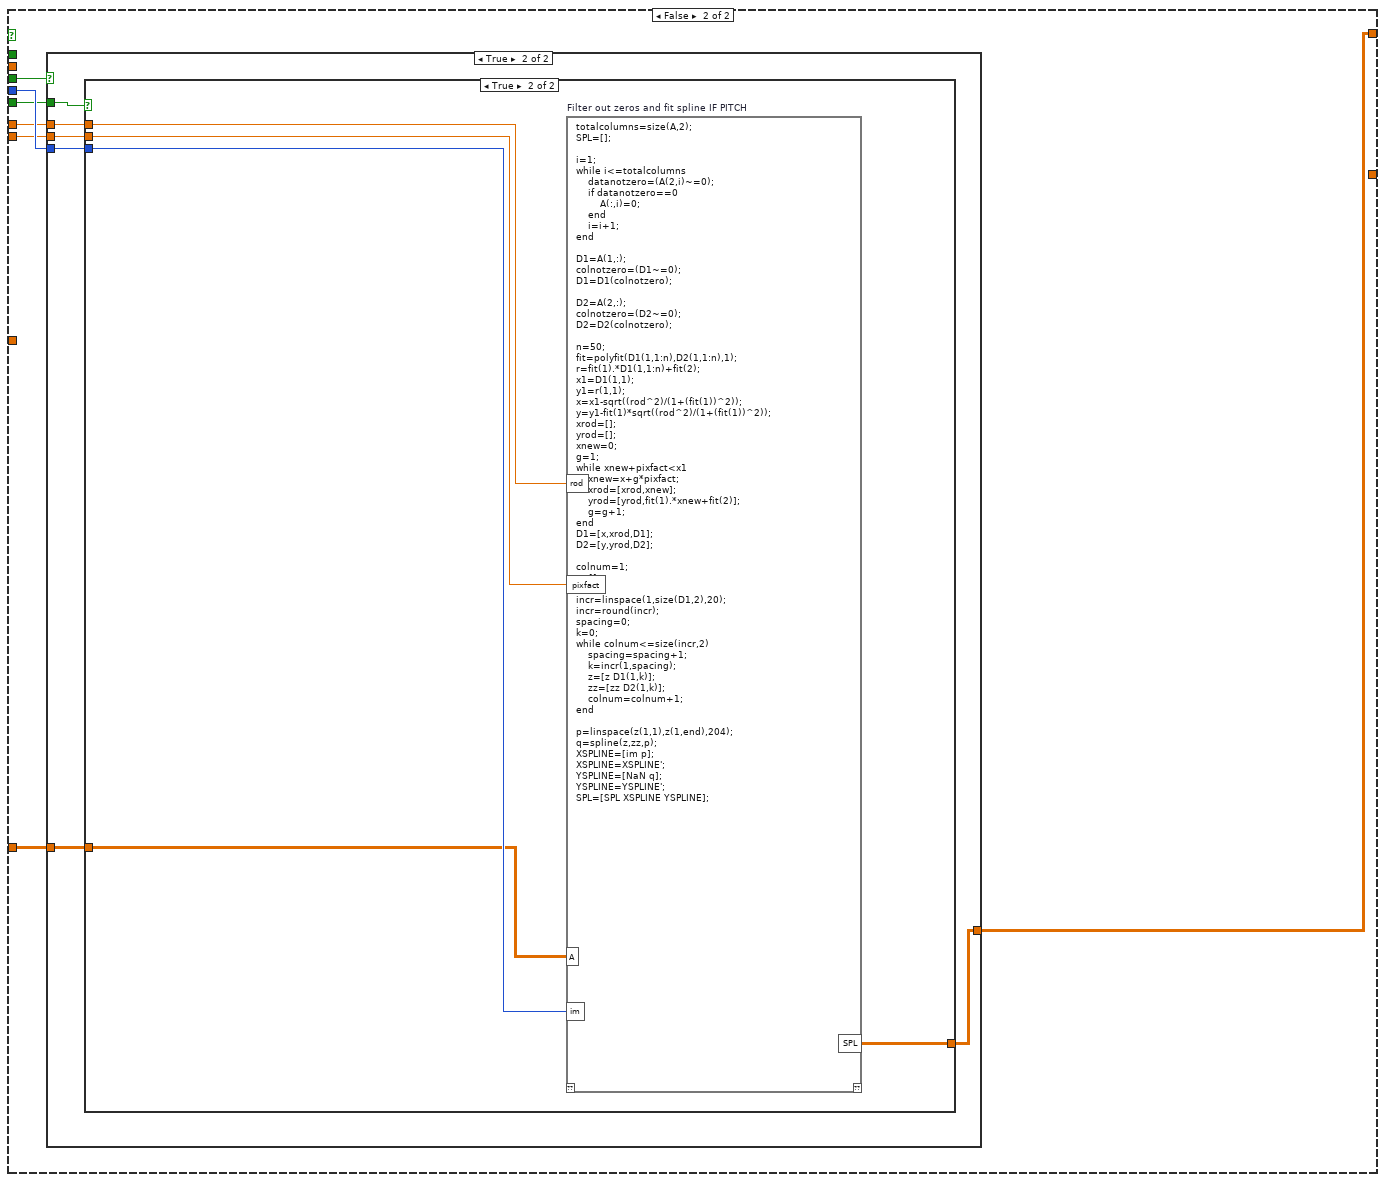
[diagram p20: hidden frame]
diagram:
  n1 = Multiply(x="Number of frames\nto analyze", y=2) -> (x*y=w32:i32)
  n2 = Multiply(x="Number of frames\nto analyze", y=2) -> (x*y=w35:i32)
  n3 = Multiply(x="Number of frames\nto analyze", y=2) -> (x*y=w15:i32)
  n4 = Initialize Array "If 2 segments, initialize\narray to store \nSNAPS splines"(0.0 ("element"), 205 ("dimension size"), w15) -> (w13:dbl[][])
  n5 = Initialize Array "Initialize Array\nto store splines"(0.0 ("element"), 205 ("dimension size"), w35) -> (w38:dbl[][])
  n6 = Initialize Array "Initialize Array\nto store raw\nsurfaces"(0.0 ("element"), w32, 1024 ("dimension size")) -> (w30:dbl[][])
  n7 = for {
    N: "Number of frames\nto analyze" -> [_]
    shift-right: [w81] -> w2
    shift-left: w38 -> [w78]
    shift-right: [w76] -> w28
    shift-left: w30 -> [w77]
    tunnel: [w56] -> w23
    tunnel: "Start frame" -> [w62]
    tunnel: "X coordinate \nwithin gap\n(in pixels)" -> [w50]
    tunnel: "Rod width (mm)" -> [w49]
    tunnel: "ON to \nsimulate rod" -> [w48]
    tunnel: "ON for 2 foil\nsegments" -> [w47]
    tunnel: "ON for pitch,\nOFF if NO pitch" -> [w46]
    shift-right: [w44] -> w1
    shift-left: w13 -> [w43]
    i -> [w53]
    w114 = T6 0 items=["Grayscale (U8)", "Grayscale (I16)", "Grayscale (SGL)", "Complex (CSG)", "RGB (U32)", "HSL (U32)", "RGB (U64)", "Grayscale (U16)"] ("Image Type")
    w118 = T6 0 items=["Grayscale (U8)", "Grayscale (I16)", "Grayscale (SGL)", "Complex (CSG)", "RGB (U32)", "HSL (U32)", "RGB (U64)", "Grayscale (U16)"] ("Image Type")
    n8 = Decrement(x=w62) -> (x-1=w61:i32)
    n9 = Add(x=w61, y=w53) -> (x+y=w60:i32)
    n10 = Increment(x=w60) -> (x+1=w80:i32)
    "current\nimage number" <- w80
    n11 = call <userlib>:"Read one image from photron AVI file.vi"("image number"=w60, "AVI file"="Foil AVI file to load") -> ("Image"=w86:T1)  [unwired: 4 in, 1 out]
    "Image" <- w86
    n12 = case shown="True" "Rotate\n90 deg (CCW)" {
      tunnel: w86 -> [w223 w226]
      tunnel: [w223 w224] -> w85
      frame False {
      }
      frame True {
        w228 = T6 0 items=["Grayscale (U8)", "Grayscale (I16)", "Grayscale (SGL)", "Complex (CSG)", "RGB (U32)", "HSL (U32)", "RGB (U64)", "Grayscale (U16)"] ("Image Type")
        n13 = call "IMAQ Create"("Image Name"="image 5", "Image Type"=w228) -> ("New Image"=w227:T1)  [unwired: 3 in, 1 out]
        n14 = call "IMAQ Rotate"("Maintain Size"=TRUE, "Angle (degrees)"=sgl 90.0, "Image Dst"=w227, "Image Src"=w226) -> ("Image Dst Out"=w224:T1)  [unwired: 6 in, 1 out]
      }
    }
    n15 = case shown="True" "Rotate\n180 deg" {
      tunnel: w85 -> [w215 w218]
      tunnel: [w215 w216] -> w67
      frame False {
      }
      frame True {
        w220 = T6 0 items=["Grayscale (U8)", "Grayscale (I16)", "Grayscale (SGL)", "Complex (CSG)", "RGB (U32)", "HSL (U32)", "RGB (U64)", "Grayscale (U16)"] ("Image Type")
        n16 = call "IMAQ Create"("Image Name"="image 6", "Image Type"=w220) -> ("New Image"=w219:T1)  [unwired: 3 in, 1 out]
        n17 = call "IMAQ Rotate"("Maintain Size"=TRUE, "Angle (degrees)"=sgl 180.0, "Image Dst"=w219, "Image Src"=w218) -> ("Image Dst Out"=w216:T1)  [unwired: 6 in, 1 out]
      }
    }
    n18 = case shown="True" "Flip along\nvertical line" {
      tunnel: w67 -> [w204 w207]
      tunnel: [w204 w206] -> w65
      frame False {
      }
      frame True {
        w205 = u32 1 items=["Horizontal", "Vertical", "Central", "1st Diagonal", "2nd Diagonal"] ("Type of Symmetry")
        w209 = T6 0 items=["Grayscale (U8)", "Grayscale (I16)", "Grayscale (SGL)", "Complex (CSG)", "RGB (U32)", "HSL (U32)", "RGB (U64)", "Grayscale (U16)"] ("Image Type")
        n19 = call "IMAQ Create"("Image Name"="image 7", "Image Type"=w209) -> ("New Image"=w208:T1)  [unwired: 3 in, 1 out]
        n20 = call "IMAQ Symmetry"("Type of Symmetry"=w205, "Image Dst"=w208, "Image Src"=w207) -> ("Image Dst Out"=w206:T1)  [unwired: 2 in, 1 out]
      }
    }
    n21 = case shown="True" "Flip along\nhorizontal line" {
      tunnel: w65 -> [w197 w200]
      tunnel: [w197 w198] -> w63
      frame False {
      }
      frame True {
        w199 = u32 0 items=["Horizontal", "Vertical", "Central", "1st Diagonal", "2nd Diagonal"] ("Type of Symmetry")
        w202 = T6 0 items=["Grayscale (U8)", "Grayscale (I16)", "Grayscale (SGL)", "Complex (CSG)", "RGB (U32)", "HSL (U32)", "RGB (U64)", "Grayscale (U16)"] ("Image Type")
        n22 = call "IMAQ Create"("Image Name"="image 8", "Image Type"=w202) -> ("New Image"=w201:T1)  [unwired: 3 in, 1 out]
        n23 = call "IMAQ Symmetry"("Type of Symmetry"=w199, "Image Dst"=w201, "Image Src"=w200) -> ("Image Dst Out"=w198:T1)  [unwired: 2 in, 1 out]
      }
    }
    "Rotated/Mirrored image" <- w63
    n24 = call "IMAQ Create"("Image Name"="image 2", "Image Type"=w118) -> ("New Image"=w121:T1)  [unwired: 3 in, 1 out]
    n25 = call "IMAQ GetImageSize"("Image"=w63) -> ("Y Resolution"=→"Y Resolution":i32, "X Resolution"=→"X Resolution":i32)  [unwired: 3 in, 1 out]
    n26 = call "IMAQ Create"("Image Name"="image 4", "Image Type"=w114) -> ("New Image"=w113:T1)  [unwired: 3 in, 1 out]
    n27 = call "IMAQ Threshold"("Replace Value"=1, "Keep/Replace Value (Replace)"=TRUE, "Range"="Range", "Image Dst"=w121, "Image Src"=w63) -> ("Image Dst Out"=w116:T1)  [unwired: 5 in, 1 out]
    n28 = call "IMAQ Create"("Image Name"="image 3") -> ("New Image"=w110:T1)  [unwired: 4 in, 1 out]
    n29 = call "IMAQ Particle Filter 3"("Image Src"=w116, "Image Dst"=w113, "Selection Values"="Selection Values", "Keep/Remove Particles (F)"=FALSE) -> ("Image Dst Out"=w105:T1)  [unwired: 9 in, 2 out]
    n30 = case shown="True" "On for\ntest display" {
      tunnel: w105 -> [_ w233]
      frame False {
      }
      frame True {
        n31 = call "IMAQ GetPalette"("Palette Number (gray)"=T5."Binary") -> ("Color Palette"=w232:cluster{"Red":u8, "Green":u8, "Blue":u8}[])  [unwired: 4 in, 1 out]
        n32 = call "IMAQ WindDraw"("Color Palette"=w232, "Image"=w233) -> ()  [unwired: 8 in, 2 out]
      }
    }
    n33 = Unbundle By Name("surface finder settings") -> ("pixel column start index"=w98:i32, "pixel column end index"=w97:i32, "analyze all\nimage\ncolumns"=w99:bool, "surface pixel offset"=w54:i32, "lowest pix intensity\nfor surface id"=w91:i32, "intensity step\nsize for search"=w92:i32, "maximum expected\nparticle width"=w94:i32, "slope of intensity\nfor surface peak id"=w93:dbl, "no body\npresent"=w100:bool, "edge position\nhigh limit"=w101:i32, "DaVis pixel\nscale factor\n(mm/pixel)"=w56:dbl)
    n34 = call "IMAQ Multiply"("Image Src A"=w63, "Image Dst"=w110, "Image Src B"=w105) -> ("Image Dst Out"=w104:T1)  [unwired: 4 in, 1 out]
    n35 = Multiply(x=w54, y=w56) -> (x*y=w51:dbl)
    n36 = Equal To 0?(x=w54) -> (x = 0?=w52:bool)
    n37 = Increment(x=w101) -> (x+1=w102:i32)
    n38 = call "IMAQ ImageToArray"("Image"=w104) -> ("Image Pixels (U8)"=w64:u8[][])  [unwired: 3 in, 4 out]
    n39 = Array Subset(array=w64, index (row)=0 ("index"), length (row)=w102) -> (w95:u8[][])  [unwired: 2 in]
    n40 = call <userlib>:"size 2D array.vi"("array in"=w95) -> ("Rows"=w90:i32, "Columns"=w96:i32)
    n41 = case shown="False" w100 {
      tunnel: w99 -> [w247 _]
      tunnel: w98 -> [w246 _]
      tunnel: w97 -> [w245 _]
      tunnel: w96 -> [w234 w323]
      tunnel: w95 -> [w242 _]
      tunnel: w94 -> [w241 _]
      tunnel: w93 -> [w240 _]
      tunnel: w92 -> [w239 _]
      tunnel: w91 -> [w238 _]
      tunnel: w54 -> [w237 _]
      tunnel: [w236 w322] -> w55
      tunnel: [w235 w325] -> w75
      tunnel: w90 -> [_ w324]
      frame False {
        n42 = case shown="False" w247 {
          tunnel: w246 -> [w318 _]
          tunnel: w245 -> [w317 _]
          tunnel: [w313 w321] -> w244
          tunnel: [w311 0] -> w243
          tunnel: w234 -> [w310 w319]
          frame False {
            n43 = Decrement(x=w310) -> (x-1=w314:i32)
            n44 = Max & Min(x=w318, y=w317) -> (max(x,y)=w315:i32, min(x,y)=w316:i32)
            n45 = Max & Min(x=w314, y=w315) -> (min(x,y)=w313:i32)  [unwired: 1 out]
            n46 = Max & Min(x=w316, y=0) -> (max(x,y)=w311:i32)  [unwired: 1 out]
          }
          frame True {
            n47 = Decrement(x=w319) -> (x-1=w321:i32)
          }
        }
        n48 = for {
          N: w234 -> [_]
          tunnel: w244 -> [w249]
          tunnel: w243 -> [w250]
          tunnel: w242 -> [w257]
          tunnel: w241 -> [w256]
          tunnel: w240 -> [w255]
          tunnel: w239 -> [w254]
          tunnel: w238 -> [w253]
          tunnel: w237 -> [w252]
          tunnel: [w251] -> w236 mode=indexing
          tunnel: [w248] -> w235 mode=indexing
          i -> [w248]
          n49 = In Range and Coerce(upper limit=w249, x=w248, lower limit=w250) -> (In Range?=w258:bool)  [unwired: 1 out]
          n50 = case shown="True" w258 {
            tunnel: w257 -> [_ w275]
            tunnel: w248 -> [_ w274]
            tunnel: w256 -> [_ w272]
            tunnel: w255 -> [_ w271]
            tunnel: w254 -> [_ w270]
            tunnel: w253 -> [_ w269]
            tunnel: w252 -> [_ w260]
            tunnel: [0 w261] -> w251
            frame False {
            }
            frame True {
              n51 = Index Array(array=w275, index (col)=w274) -> (element=w266:u8[])  [unwired: 1 in]
              n52 = Array Size(array=w266) -> (size(s)=w267:i32)
              n53 = Array Max & Min(array=w266) -> (max value=w273:u8)  [unwired: 3 out]
              n54 = while {
                tunnel: w274 -> [_]
                tunnel: w266 -> [w295]
                shift-right: [w287] -> _
                shift-left: w273 -> [w282]
                tunnel: w272 -> [w293]
                tunnel: w271 -> [w292]
                shift-right: [w283] -> _
                shift-left: w270 -> [w284]
                tunnel: w269 -> [w281]
                tunnel: [w279] -> w261
                stop <- w291 stop-if-true
                n55 = Less?(x=w282, y=w281) -> (x < y?=w280:bool)
                n56 = Subtract(x=w282, y=w284) -> (x-y=w288:i32)
                n57 = Not Equal?(x=w284, y=1) -> (x != y?=w289:bool)
                n58 = Equal?(x=w284, y=1) -> (x = y?=w277:bool)
                n59 = case shown="False" "use max\npixel for \nsurface" {
                  tunnel: w295 -> [w307 w309]
                  tunnel: [w303 w308] -> w279
                  tunnel: w282 -> [w306 _]
                  tunnel: w293 -> [w305 _]
                  tunnel: w292 -> [w304 _]
                  frame False {
                    n60 = call <userlib>:"vector edge finder.vi"("slope threshold"=w304, "width"=w305, "threshold"=w306, "vector"=w307) -> ("first edge pixel"=w303:i32)  [unwired: 1 out]
                  }
                  frame True {
                    n61 = Array Max & Min(array=w309) -> (max index (indices)=w308:i32)  [unwired: 3 out]
                  }
                }
                n62 = Not Equal To 0?(x=w279) -> (x != 0?=w276:bool)
                n63 = And(x=w276, y=w277) -> (x .and. y?=w278:bool)
                n64 = And(x=w276, y=w289) -> (x .and. y?=w290:bool)
                n65 = Or(x=w278, y=w280) -> (x .or. y?=w291:bool)
                n66 = case shown="True" w290 {
                  tunnel: w288 -> [w296 w302]
                  tunnel: [w296 w300] -> w287
                  tunnel: w284 -> [_ w299]
                  tunnel: w284 -> [w297 _]
                  tunnel: [w297 1] -> w283
                  frame False {
                  }
                  frame True {
                    n67 = Add(x=w302, y=w299) -> (x+y=w301:i32)
                    n68 = Decrement(x=w301) -> (x-1=w300:i32)
                  }
                }
              }
              n69 = Add(x=w261, y=w260) -> (x+y=w263:i32)
              n70 = Initialize Array(0 ("element"), w267) -> (w268:i32[])
              n71 = Replace Array Subset(array=w268, new element=255 ("new element/subarray"), index=w263) -> (w265:i32[])
              n72 = Build Cluster Array(w266, w265) -> ()  [unwired: 1 out]
            }
          }
        }
      }
      frame True {
        n73 = Initialize Array(w324, w323) -> (w322:i32[])
        n74 = for {
          N: w323 -> [_]
          tunnel: [w326] -> w325 mode=indexing
          i -> [w326]
        }
      }
    }
    n75 = Build Cluster Array(w75, w55) -> (→"surface":cluster{i32, "Rows":i32}[])
    n76 = Build Array(w75) -> (w74:i32[][])
    n77 = Build Array(w55) -> (w73:i32[][])
    n78 = script code="A=[X;Y];\ntotalcolumns=size(A,2);\n\ni=1;\nwhile i<=totalcolumns\n    dataneg=(A(2,i)<0);\n    if dataneg==1\n        A(2,i)=0;\n    end\n    i=i+1;\nend" "Get rid of any negative values (error values)"("X"=w74, "Y"=w73) -> ("A"=w59:dbl[][])  [unwired: 1 in, 1 out]
    n79 = Multiply(x=w59, y=w56) -> (x*y=w71:dbl[][])
    n80 = case shown="False" "For raw detected\nsurface:\nOn for mm,\nOff for pixels" {
      tunnel: w59 -> [w211 w213]
      tunnel: [w211 w214] -> w70
      tunnel: w56 -> [_ w212]
      frame False {
      }
      frame True {
        n81 = Multiply(x=w212, y=w213) -> (x*y=w214:dbl[][])
      }
    }
    n82 = case shown="True" w47 {
      tunnel: w80 -> [w129 w173]
      tunnel: w71 -> [w131 w172]
      tunnel: w48 -> [w134 w171]
      tunnel: [w127 w170] -> w58
      tunnel: w56 -> [w128 w169]
      tunnel: w46 -> [w133 w168]
      tunnel: w49 -> [w132 w167]
      tunnel: w50 -> [w130 _]
      tunnel: w52 -> [w125 _]
      tunnel: w51 -> [w124 _]
      tunnel: [w123 _] -> w45
      frame True {
        n83 = case shown="False" w134 {
          tunnel: w133 -> [_ w152]
          tunnel: w132 -> [_ w151]
          tunnel: w131 -> [w144 w150]
          tunnel: w130 -> [w141 w149]
          tunnel: w129 -> [w142 w148]
          tunnel: w128 -> [w143 w147]
          tunnel: [w140 w146] -> w127
          tunnel: [w139 w145] -> w126
          frame False {
            n84 = script code="Afront = [];\nAback = [];\n\nn=1;\nwhile n<gapx\n    Afront(:,n) = A(:,n);\n    n = n+1;\n    \nend\n\nback_index = 1;\nwhile n < 1025;\n    Aback(:,back_index)=A(:,n);\n    n = n+1;\n    back_index=back_index+1;\n    \nend\n\n\ntotcolf = size(Afront,2);\n\ni=1;        \nwhile i<=totcolf\n    datanotzero=(Afront(2,i)~=0);\n    if datanotzero==0\n        Afront(:,i)=0;\n    end\n    i=i+1;\nend\n\n\nD1f=Afront(1,:);\ncolnotzero=(D1f~=0);\nD1f=D1f(colnotzero);\n\nD2f=Afront(2,:);\ncolnotzero=(D2f~=0);\nD2f=D2f(colnotzero);\n\n\n \n\ncolnum=1;\nzf=[];\nzzf=[];\nincr=linspace(1,size(D1f,2),20);\nincr=round(incr);\nspacing=0;\nk=0;\nwhile colnum<=size(incr,2)\n    spacing=spacing+1;\n    k=incr(1,spacing);\n    zf=[zf D1f(1,k)];\n    zzf=[zzf D2f(1,k)];\n    colnum=colnum+1;\nend\n\npf=linspace(zf(1,1),zf(1,end),104);\nqf=spline(zf,zzf,pf);\nXSPLINEf=[im pf];\nXSPLINEf=XSPLINEf';\nYSPLINEf=[NaN qf];\nYSPLINEf=YSPLINEf';\nSPLf=[XSPLINEf YSPLINEf];\n\n\n\ntotcolb = size(Aback,2);\n\ni=1;\nwhile i<=totcolb\n    datanotzero=(Aback(2,i)~=0);\n    if datanotzero==0\n        Aback(:,i)=0;\n    end\n    i=i+1;\nend\n\nD1b=Aback(1,:);\ncolnotzero=(D1b~=0);\nD1b=D1b(colnotzero);\n\nD2b=Aback(2,:);\ncolnotzero=(D2b~=0);\nD2b=D2b(colnotzero);\n\n\n\ncolnum=1;\nzb=[];\nzzb=[];\nincr=linspace(1,size(D1b,2),20);\nincr=round(incr);\nspacing=0;\nk=0;\nwhile colnum<=size(incr,2)\n    spacing=spacing+1;\n    k=incr(1,spacing);\n    zb=[zb D1b(1,k)];\n    zzb=[zzb D2b(1,k)];\n    colnum=colnum+1;\nend\n\npb=linspace(zb(1,1),zb(1,end),100);\nqb=spline(zb,zzb,pb);\nXSPLINEb=[pb];         \nXSPLINEb=XSPLINEb';\nYSPLINEb=[qb];        \nYSPLINEb=YSPLINEb';\nSPLb=[XSPLINEb YSPLINEb];\n\n\n\nSPL=[SPLf;SPLb];\n\n\npf_snaps = linspace(zf(1,1),zf(1,end),size(D1f,2));\nqf_snaps = spline(zf,zzf,pf_snaps);\n\npb_snaps = linspace(zb(1,1),zb(1,end),size(D1b,2));\nqb_snaps = spline(zb,zzb,pb_snaps);\n\n\nxsnapsf=[pf_snaps];         \nxsnapsf=xsnapsf';\nysnapsf=[qf_snaps];        \nysnapsf=ysnapsf';\nsnapsf = [xsnapsf ysnapsf];\n\n\nxsnapsb=[pb_snaps];         \nxsnapsb=xsnapsb';\nysnapsb=[qb_snaps];        \nysnapsb=ysnapsb';\nsnapsb = [xsnapsb ysnapsb];\n\n\nTEfx = max(xsnapsf);\nLEbx = xsnapsb(1);\n\n\nallXvals = A(1,:);\n\n[tf, indTEf] = ismember(TEfx, allXvals);\n[tf, indLEb] = ismember(LEbx, allXvals);\n\n\ngap_xcoor = [];\n\n\ncol = indTEf+1;\nn=1;\n\n\nwhile col < indLEb\n    \n    gap_xcoor(n) = allXvals(col);\n    col = col + 1;\n    n = n+1;\n    \nend\n\n\n\ngap_ycoor = zeros(size(gap_xcoor,2),1);\ngap_xcoor = gap_xcoor';\ngap_coor = [gap_xcoor gap_ycoor];\n\nallPix = [snapsf; gap_coor; snapsb];\n\n\nSNAPSx = [];\nSNAPSy = [];\n\n\ncolnum = 1;\nincr=linspace(1,size(allPix,1),204);\nincr=round(incr);\nspacing=0;\nk=0;\nwhile colnum<=size(incr,2)\n    spacing=spacing+1;\n    k=incr(1,spacing);\n    SNAPSx=[SNAPSx allPix(k,1)];\n    SNAPSy=[SNAPSy allPix(k,2)];\n    colnum=colnum+1;\nend\n\nSNAPSx = [im SNAPSx];\nSNAPSx = SNAPSx';\nSNAPSy = [NaN SNAPSy];\nSNAPSy = SNAPSy';\nSNAPS = [SNAPSx SNAPSy];" "2 segments, NO rod sim"("A"=w144, "pixfact"=w143, "im"=w142, "gapx"=w141) -> ("SPL"=w140:dbl[][], "SNAPS"=w139:dbl[][])  [unwired: 1 in, 1 out]
          }
          frame True {
            n85 = case shown="True" w152 {
              tunnel: w151 -> [w158 w166]
              tunnel: w150 -> [w159 w165]
              tunnel: w149 -> [w156 w164]
              tunnel: w148 -> [w157 w163]
              tunnel: w147 -> [w155 w162]
              tunnel: [w154 w161] -> w146
              tunnel: [w153 w160] -> w145
              frame False {
                n86 = script code="Afront = [];\nAback = [];\n\nn=1;\nwhile n<gapx\n    Afront(:,n) = A(:,n);\n    n = n+1;\n    \nend\n\nback_index = 1;\nwhile n < 1025;\n    Aback(:,back_index)=A(:,n);\n    n = n+1;\n    back_index=back_index+1;\n    \nend\n\n\ntotcolf = size(Afront,2);\n\ni=1;        \nwhile i<=totcolf\n    datanotzero=(Afront(2,i)~=0);\n    if datanotzero==0\n        Afront(:,i)=0;\n    end\n    i=i+1;\nend\n\n\nD1f=Afront(1,:);\ncolnotzero=(D1f~=0);\nD1f=D1f(colnotzero);\n\nD2f=Afront(2,:);\ncolnotzero=(D2f~=0);\nD2f=D2f(colnotzero);\n\n\n \nx1f=D1f(1,1);\ny1f=mean(D2f(1,1:10));\nxf=x1f-rod;\nyf=y1f;\nxrod=[];\nyrod=[];\nxnew=0;\ng=1;\nwhile xnew+pixfact<x1f\n    xnew=xf+g*pixfact;\n    xrod=[xrod,xnew];\n    yrod=[yrod,y1f];\n    g=g+1;\nend\nD1f=[xf,xrod,D1f];\nD2f=[yf,yrod,D2f];\n\n\n\ncolnum=1;\nzf=[];\nzzf=[];\nincr=linspace(1,size(D1f,2),20);\nincr=round(incr);\nspacing=0;\nk=0;\nwhile colnum<=size(incr,2)\n    spacing=spacing+1;\n    k=incr(1,spacing);\n    zf=[zf D1f(1,k)];\n    zzf=[zzf D2f(1,k)];\n    colnum=colnum+1;\nend\n\npf=linspace(zf(1,1),zf(1,end),104);\nqf=spline(zf,zzf,pf);\nXSPLINEf=[im pf];\nXSPLINEf=XSPLINEf';\nYSPLINEf=[NaN qf];\nYSPLINEf=YSPLINEf';\nSPLf=[XSPLINEf YSPLINEf];\n\n\n\ntotcolb = size(Aback,2);\n\ni=1;\nwhile i<=totcolb\n    datanotzero=(Aback(2,i)~=0);\n    if datanotzero==0\n        Aback(:,i)=0;\n    end\n    i=i+1;\nend\n\nD1b=Aback(1,:);\ncolnotzero=(D1b~=0);\nD1b=D1b(colnotzero);\n\nD2b=Aback(2,:);\ncolnotzero=(D2b~=0);\nD2b=D2b(colnotzero);\n\n\n\ncolnum=1;\nzb=[];\nzzb=[];\nincr=linspace(1,size(D1b,2),20);\nincr=round(incr);\nspacing=0;\nk=0;\nwhile colnum<=size(incr,2)\n    spacing=spacing+1;\n    k=incr(1,spacing);\n    zb=[zb D1b(1,k)];\n    zzb=[zzb D2b(1,k)];\n    colnum=colnum+1;\nend\n\npb=linspace(zb(1,1),zb(1,end),100);\nqb=spline(zb,zzb,pb);\nXSPLINEb=[pb];         \nXSPLINEb=XSPLINEb';\nYSPLINEb=[qb];        \nYSPLINEb=YSPLINEb';\nSPLb=[XSPLINEb YSPLINEb];\n\n\n\nSPL=[SPLf;SPLb];\n\n\npf_snaps = linspace(zf(1,1),zf(1,end),size(D1f,2));\nqf_snaps = spline(zf,zzf,pf_snaps);\n\npb_snaps = linspace(zb(1,1),zb(1,end),size(D1b,2));\nqb_snaps = spline(zb,zzb,pb_snaps);\n\n\nxsnapsf=[pf_snaps];         \nxsnapsf=xsnapsf';\nysnapsf=[qf_snaps];        \nysnapsf=ysnapsf';\nsnapsf = [xsnapsf ysnapsf];\n\n\nxsnapsb=[pb_snaps];         \nxsnapsb=xsnapsb';\nysnapsb=[qb_snaps];        \nysnapsb=ysnapsb';\nsnapsb = [xsnapsb ysnapsb];\n\n\nTEfx = max(xsnapsf);\nLEbx = xsnapsb(1);\n\n\nallXvals = A(1,:);\n\n[tf, indTEf] = ismember(TEfx, allXvals);\n[tf, indLEb] = ismember(LEbx, allXvals);\n\n\ngap_xcoor = [];\n\n\ncol = indTEf+1;\nn=1;\n\n\nwhile col < indLEb\n    \n    gap_xcoor(n) = allXvals(col);\n    col = col + 1;\n    n = n+1;\n    \nend\n\n\n\ngap_ycoor = zeros(size(gap_xcoor,2),1);\ngap_xcoor = gap_xcoor';\ngap_coor = [gap_xcoor gap_ycoor];\n\nallPix = [snapsf; gap_coor; snapsb];\n\n\nSNAPSx = [];\nSNAPSy = [];\n\n\ncolnum = 1;\nincr=linspace(1,size(allPix,1),204);\nincr=round(incr);\nspacing=0;\nk=0;\nwhile colnum<=size(incr,2)\n    spacing=spacing+1;\n    k=incr(1,spacing);\n    SNAPSx=[SNAPSx allPix(k,1)];\n    SNAPSy=[SNAPSy allPix(k,2)];\n    colnum=colnum+1;\nend\n\nSNAPSx = [im SNAPSx];\nSNAPSx = SNAPSx';\nSNAPSy = [NaN SNAPSy];\nSNAPSy = SNAPSy';\nSNAPS = [SNAPSx SNAPSy];" "2 segments, sim rod NO pitch"("A"=w159, "im"=w157, "rod"=w158, "pixfact"=w155, "gapx"=w156) -> ("SPL"=w154:dbl[][], "SNAPS"=w153:dbl[][])  [unwired: 1 in, 1 out]
              }
              frame True {
                n87 = script code="Afront = [];\nAback = [];\n\nn=1;\nwhile n<gapx\n    Afront(:,n) = A(:,n);\n    n = n+1;\n    \nend\n\nback_index = 1;\nwhile n < 1025;\n    Aback(:,back_index)=A(:,n);\n    n = n+1;\n    back_index=back_index+1;\n    \nend\n\n\ntotcolf = size(Afront,2);\n\ni=1;        \nwhile i<=totcolf\n    datanotzero=(Afront(2,i)~=0);\n    if datanotzero==0\n        Afront(:,i)=0;\n    end\n    i=i+1;\nend\n\n\nD1f=Afront(1,:);\ncolnotzero=(D1f~=0);\nD1f=D1f(colnotzero);\n\nD2f=Afront(2,:);\ncolnotzero=(D2f~=0);\nD2f=D2f(colnotzero);\n\n\n\nn=50;\nfit=polyfit(D1f(1,1:n),D2f(1,1:n),1);\nr=fit(1).*D1f(1,1:n)+fit(2);\nx1=D1f(1,1);\ny1=r(1,1);\nx=x1-sqrt((rod^2)/(1+(fit(1))^2));\ny=y1-fit(1)*sqrt((rod^2)/(1+(fit(1))^2));\nxrod=[];\nyrod=[];\nxnew=0;\ng=1;\nwhile xnew+pixfact<x1\n    xnew=x+g*pixfact;\n    xrod=[xrod,xnew];\n    yrod=[yrod,fit(1).*xnew+fit(2)];\n    g=g+1;\nend\nD1f=[x,xrod,D1f];\nD2f=[y,yrod,D2f];\n\n\n\ncolnum=1;\nzf=[];\nzzf=[];\nincr=linspace(1,size(D1f,2),20);\nincr=round(incr);\nspacing=0;\nk=0;\nwhile colnum<=size(incr,2)\n    spacing=spacing+1;\n    k=incr(1,spacing);\n    zf=[zf D1f(1,k)];\n    zzf=[zzf D2f(1,k)];\n    colnum=colnum+1;\nend\n\npf=linspace(zf(1,1),zf(1,end),104);\nqf=spline(zf,zzf,pf);\nXSPLINEf=[im pf];\nXSPLINEf=XSPLINEf';\nYSPLINEf=[NaN qf];\nYSPLINEf=YSPLINEf';\nSPLf=[XSPLINEf YSPLINEf];\n\n\n\ntotcolb = size(Aback,2);\n\ni=1;\nwhile i<=totcolb\n    datanotzero=(Aback(2,i)~=0);\n    if datanotzero==0\n        Aback(:,i)=0;\n    end\n    i=i+1;\nend\n\nD1b=Aback(1,:);\ncolnotzero=(D1b~=0);\nD1b=D1b(colnotzero);\n\nD2b=Aback(2,:);\ncolnotzero=(D2b~=0);\nD2b=D2b(colnotzero);\n\n\n\ncolnum=1;\nzb=[];\nzzb=[];\nincr=linspace(1,size(D1b,2),20);\nincr=round(incr);\nspacing=0;\nk=0;\nwhile colnum<=size(incr,2)\n    spacing=spacing+1;\n    k=incr(1,spacing);\n    zb=[zb D1b(1,k)];\n    zzb=[zzb D2b(1,k)];\n    colnum=colnum+1;\nend\n\npb=linspace(zb(1,1),zb(1,end),100);\nqb=spline(zb,zzb,pb);\nXSPLINEb=[pb];         \nXSPLINEb=XSPLINEb';\nYSPLINEb=[qb];        \nYSPLINEb=YSPLINEb';\nSPLb=[XSPLINEb YSPLINEb];\n\n\n\nSPL=[SPLf;SPLb];\n\n\npf_snaps = linspace(zf(1,1),zf(1,end),size(D1f,2));\nqf_snaps = spline(zf,zzf,pf_snaps);\n\npb_snaps = linspace(zb(1,1),zb(1,end),size(D1b,2));\nqb_snaps = spline(zb,zzb,pb_snaps);\n\n\nxsnapsf=[pf_snaps];         \nxsnapsf=xsnapsf';\nysnapsf=[qf_snaps];        \nysnapsf=ysnapsf';\nsnapsf = [xsnapsf ysnapsf];\n\n\nxsnapsb=[pb_snaps];         \nxsnapsb=xsnapsb';\nysnapsb=[qb_snaps];        \nysnapsb=ysnapsb';\nsnapsb = [xsnapsb ysnapsb];\n\n\nTEfx = max(xsnapsf);\nLEbx = xsnapsb(1);\n\n\nallXvals = A(1,:);\n\n[tf, indTEf] = ismember(TEfx, allXvals);\n[tf, indLEb] = ismember(LEbx, allXvals);\n\n\ngap_xcoor = [];\n\n\ncol = indTEf+1;\nn=1;\n\n\nwhile col < indLEb\n    \n    gap_xcoor(n) = allXvals(col);\n    col = col + 1;\n    n = n+1;\n    \nend\n\n\n\ngap_ycoor = zeros(size(gap_xcoor,2),1);\ngap_xcoor = gap_xcoor';\ngap_coor = [gap_xcoor gap_ycoor];\n\nallPix = [snapsf; gap_coor; snapsb];\n\n\nSNAPSx = [];\nSNAPSy = [];\n\n\ncolnum = 1;\nincr=linspace(1,size(allPix,1),204);\nincr=round(incr);\nspacing=0;\nk=0;\nwhile colnum<=size(incr,2)\n    spacing=spacing+1;\n    k=incr(1,spacing);\n    SNAPSx=[SNAPSx allPix(k,1)];\n    SNAPSy=[SNAPSy allPix(k,2)];\n    colnum=colnum+1;\nend\n\nSNAPSx = [im SNAPSx];\nSNAPSx = SNAPSx';\nSNAPSy = [NaN SNAPSy];\nSNAPSy = SNAPSy';\nSNAPS = [SNAPSx SNAPSy];" "2 segments, sim rod with pitch"("A"=w165, "rod"=w166, "pixfact"=w162, "im"=w163, "gapx"=w164) -> ("SPL"=w161:dbl[][], "SNAPS"=w160:dbl[][])  [unwired: 1 in, 1 out]
              }
            }
          }
        }
        n88 = case "Optionally add in pixel offset value\n(for thick foils)" shown="False" w125 {
          tunnel: w126 -> [w137 w138]
          tunnel: [w136 w138] -> w123
          tunnel: w124 -> [w135 _]
          frame False {
            n89 = script code="i=2;\nwhile i<=size(SNAPS,2)\n    SNAPS(2:end,i)=SNAPS(2:end,i)+offset;\n    i=i+2;\nend"("SNAPS"=w137, "offset"=w135) -> ("SNAPS"=w136:dbl[][])  [unwired: 1 in, 1 out]
          }
          frame True {
          }
        }
      }
      frame False {
        n90 = case shown="True" w171 {
          tunnel: w173 -> [w174 w182]
          tunnel: [w175 w181] -> w170
          tunnel: w172 -> [w176 w180]
          tunnel: w169 -> [_ w179]
          tunnel: w168 -> [_ w178]
          tunnel: w167 -> [_ w177]
          frame False {
            n91 = script code="totalcolumns=size(A,2);\nSPL=[];\n\ni=1;\nwhile i<=totalcolumns\n    datanotzero=(A(2,i)~=0);\n    if datanotzero==0\n        A(:,i)=0;\n    end\n    i=i+1;\nend\n\nD1=A(1,:);\ncolnotzero=(D1~=0);\nD1=D1(colnotzero);\n\nD2=A(2,:);\ncolnotzero=(D2~=0);\nD2=D2(colnotzero);\n\ncolnum=1;\nz=[];\nzz=[];\nincr=linspace(1,size(D1,2),20);\nincr=round(incr);\nspacing=0;\nk=0;\nwhile colnum<=size(incr,2)\n    spacing=spacing+1;\n    k=incr(1,spacing);\n    z=[z D1(1,k)];\n    zz=[zz D2(1,k)];\n    colnum=colnum+1;\nend\n\np=linspace(z(1,1),z(1,end),204);\nq=spline(z,zz,p);\nXSPLINE=[im p];\nXSPLINE=XSPLINE';\nYSPLINE=[NaN q];\nYSPLINE=YSPLINE';\n\nSPL=[XSPLINE YSPLINE]" "Filter out zeros and fit spline - ROD IS DETECTED"("A"=w176, "im"=w174) -> ("SPL"=w175:dbl[][])  [unwired: 1 in, 1 out]
          }
          frame True {
            n92 = case shown="True" w178 {
              tunnel: w182 -> [w186 w192]
              tunnel: [w185 w191] -> w181
              tunnel: w180 -> [w187 w190]
              tunnel: w177 -> [w183 w189]
              tunnel: w179 -> [w184 w188]
              frame False {
                n93 = script code="totalcolumns=size(A,2);\nSPL=[];\n\ni=1;\nwhile i<=totalcolumns\n    datanotzero=(A(2,i)~=0);\n    if datanotzero==0\n        A(:,i)=0;\n    end\n    i=i+1;\nend\n\nD1=A(1,:);\ncolnotzero=(D1~=0);\nD1=D1(colnotzero);\n\nD2=A(2,:);\ncolnotzero=(D2~=0);\nD2=D2(colnotzero);\n\nx1=D1(1,1);\ny1=mean(D2(1,1:10));\nx=x1-rod;\ny=y1;\nxrod=[];\nyrod=[];\nxnew=0;\ng=1;\nwhile xnew+pixfact<x1\n    xnew=x+g*pixfact;\n    xrod=[xrod,xnew];\n    yrod=[yrod,y1];\n    g=g+1;\nend\nD1=[x,xrod,D1];\nD2=[y,yrod,D2];\n\ncolnum=1;\nz=[];\nzz=[];\nincr=linspace(1,size(D1,2),20);\nincr=round(incr);\nspacing=0;\nk=0;\nwhile colnum<=size(incr,2)\n    spacing=spacing+1;\n    k=incr(1,spacing);\n    z=[z D1(1,k)];\n    zz=[zz D2(1,k)];\n    colnum=colnum+1;\nend\n\np=linspace(z(1,1),z(1,end),204);\nq=spline(z,zz,p);\nXSPLINE=[im p];\nXSPLINE=XSPLINE';\nYSPLINE=[NaN q];\nYSPLINE=YSPLINE';\nSPL=[XSPLINE YSPLINE];" "Filter out zeros and fit spline WITHOUT PITCH"("A"=w187, "im"=w186, "rod"=w183, "pixfact"=w184) -> ("SPL"=w185:dbl[][])  [unwired: 1 in, 1 out]
              }
              frame True {
                n94 = script code="totalcolumns=size(A,2);\nSPL=[];\n\ni=1;\nwhile i<=totalcolumns\n    datanotzero=(A(2,i)~=0);\n    if datanotzero==0\n        A(:,i)=0;\n    end\n    i=i+1;\nend\n\nD1=A(1,:);\ncolnotzero=(D1~=0);\nD1=D1(colnotzero);\n\nD2=A(2,:);\ncolnotzero=(D2~=0);\nD2=D2(colnotzero);\n\nn=50;\nfit=polyfit(D1(1,1:n),D2(1,1:n),1);\nr=fit(1).*D1(1,1:n)+fit(2);\nx1=D1(1,1);\ny1=r(1,1);\nx=x1-sqrt((rod^2)/(1+(fit(1))^2));\ny=y1-fit(1)*sqrt((rod^2)/(1+(fit(1))^2));\nxrod=[];\nyrod=[];\nxnew=0;\ng=1;\nwhile xnew+pixfact<x1\n    xnew=x+g*pixfact;\n    xrod=[xrod,xnew];\n    yrod=[yrod,fit(1).*xnew+fit(2)];\n    g=g+1;\nend\nD1=[x,xrod,D1];\nD2=[y,yrod,D2];\n\ncolnum=1;\nz=[];\nzz=[];\nincr=linspace(1,size(D1,2),20);\nincr=round(incr);\nspacing=0;\nk=0;\nwhile colnum<=size(incr,2)\n    spacing=spacing+1;\n    k=incr(1,spacing);\n    z=[z D1(1,k)];\n    zz=[zz D2(1,k)];\n    colnum=colnum+1;\nend\n\np=linspace(z(1,1),z(1,end),204);\nq=spline(z,zz,p);\nXSPLINE=[im p];\nXSPLINE=XSPLINE';\nYSPLINE=[NaN q];\nYSPLINE=YSPLINE';\nSPL=[SPL XSPLINE YSPLINE];" "Filter out zeros and fit spline IF PITCH"("A"=w190, "im"=w192, "rod"=w189, "pixfact"=w188) -> ("SPL"=w191:dbl[][])  [unwired: 1 in, 1 out]
              }
            }
          }
        }
      }
    }
    n95 = case "Optionally add in pixel offset value\n(for thick foils)" shown="False" w52 {
      tunnel: w58 -> [w195 w196]
      tunnel: [w194 w196] -> w57
      tunnel: w51 -> [w193 _]
      frame False {
        n96 = script code="i=2;\nwhile i<=size(SPL,2)\n    SPL(2:end,i)=SPL(2:end,i)+offset;\n    i=i+2;\nend"("SPL"=w195, "offset"=w193) -> ("SPL"=w194:dbl[][])  [unwired: 1 in, 1 out]
      }
      frame True {
      }
    }
    n97 = Multiply(x=2, y=w53) -> (x*y=w41:i32)
    n98 = Replace Array Subset "Store raw\nsurfaces"(array=w77, new element=w70, index (row)=w41, index (col)=0 ("disabled index (col)")) -> (w76:dbl[][])
    n99 = Replace Array Subset "Store splines"(array=w78, new element=w57, index (row)=0, index (col)=w41) -> (w81:dbl[][])
    n100 = Replace Array Subset "Store SNAPS"(array=w43, new element=w45, index (row)=0 ("disabled index (col)"), index (col)=w41) -> (w44:dbl[][])
  }
  n101 = Divide "Frames/cycle"(x="Number of frames\nto analyze", y="Number of\ncycles") -> (x/y=w26:dbl)
  n102 = call <userlib>:"size 2D array.vi"("array in"=w2) -> ("Rows"=w4:i32, "Columns"=w3:i32)
  n103 = call <userlib>:"size 2D array.vi"("array in"=w1) -> ("Rows"=w6:i32, "Columns"=w5:i32)
  n104 = case shown="True" "Save raw \ndetected\nsurface to\nspreadsheet" {
    tunnel: w28 -> [_ w328]
    frame False {
    }
    frame True {
      n105 = call-poly <vilib>:"Write To Spreadsheet File.vi"("2D data"=w328, "file path (dialog if empty)"="File path for surfaces (dialog if empty)") -> ()  [unwired: 6 in, 1 out]
    }
  }
  n106 = case shown="True" "Save an avi\nanimation" {
    tunnel: w2 -> [_ w337]
    tunnel: w23 -> [_ w330]
    tunnel: "ON for 2 foil\nsegments" -> [_ w333]
    tunnel: "X coordinate \nwithin gap\n(in pixels)" -> [_ w332]
    tunnel: w1 -> [_ w329]
    frame False {
    }
    frame True {
      n107 = Multiply(x=w332, y=w330) -> (x*y=w331:dbl)
      n108 = Multiply(x=1024, y=w330) -> (x*y=w335:dbl)
      n109 = Path To String(path="File path for kinematics avi") -> (string=w338:string)
      n110 = case shown="True" w333 {
        tunnel: w338 -> [w343 w350]
        tunnel: w337 -> [_ w349]
        tunnel: w335 -> [w345 w348]
        tunnel: "Frame increment\nfor kinematics avi" -> [w346 w347]
        tunnel: w331 -> [w344 _]
        tunnel: w329 -> [w340 _]
        frame True {
          n111 = Add(x=w340, y=0) -> (x+y=w342:dbl[][])
          n112 = script code="j=0;\nimagenum=1;\nc1=1;\nc2=2;\nSPLINES=preSPLINES(2:end,:);\nclear M\n\n\nwhile imagenum<=size(SPLINES,2)/2\n    \n    p=SPLINES(:,c1);\n    q=SPLINES(:,c2);\n    \n    ind = 1;\n    \n    while ind < size(q,1)+1\n        if q(ind) ~= 0\n            q(ind)= Scale - q(ind);\n        end\n        ind = ind + 1;\n    end\n    \n    \n\n    pfront = [];\n    qfront = [];\n    n = 1;\n    \n\n    [tf, num]=ismember(round(gapx),round(p));\n\n\n    while n<num\n        pfront = [pfront, p(n)];\n        qfront = [qfront, q(n)];\n        n=n+1;\n    end\n\n\n    pback = [];\n    qback = [];\n\n\n    while n < size(p,1)+1\n        pback = [pback, p(n)];\n        qback = [qback, q(n)];\n        n=n+1;\n    end\n\n\n    totcol = size(pfront,2);\n    i=1;\n    while i<=totcol\n        datanotzero=(qfront(1,i)~=0);\n        if datanotzero==0\n            pfront(1,i)=0;\n        end\n        i=i+1;\n    end\n\n\n    totcol = size(pback,2);\n    i=1;\n    while i<=totcol\n        datanotzero=(qback(1,i)~=0);\n        if datanotzero==0\n            pback(1,i)=0;\n        end\n        i=i+1;\n    end\n\n\n    pfront=pfront(1,:);\n    colnotzero=(pfront~=0);\n    pfront=pfront(colnotzero);\n\n    qfront=qfront(1,:);\n    colnotzero=(qfront~=0);\n    qfront=qfront(colnotzero);\n\n    pback=pback(1,:);\n    colnotzero=(pback~=0);\n    pback=pback(colnotzero);\n\n    qback=qback(1,:);\n    colnotzero=(qback~=0);\n    qback=qback(colnotzero);\n\n\n    figure(1)\n    plot(pfront,qfront,'Color',[0,0.4470,0.7410],'LineWidth',2)\n    hold on\n    plot(pback,qback,'Color',[0,0.4470,0.7410],'LineWidth',2)\n    axis([0 Scale 0 Scale])\n    hold off\n    \n    \n    \n\n    j=j+1;\n    M(j)=getframe(gcf);\n    \n    \n    c1=c1+2*Step;\n    c2=c2+2*Step;\n\n    imagenum=imagenum+Step;\n\nend\n    \nmovie2avi(M,F)"("gapx"=w344, "preSPLINES"=w342, "Step"=w346, "F"=w343, "Scale"=w345) -> ()  [unwired: 1 in, 1 out]
        }
        frame False {
          n113 = script code="j=0;\nimagenum=1;\nc1=1;\nc2=2;\nSPLINES=preSPLINES(2:end,:);\nclear M\n\n\nwhile imagenum<=size(SPLINES,2)/2\n    \n    p=SPLINES(:,c1);\n    q=SPLINES(:,c2);\n    q=Scale-q;\n\n    figure(1)\n    plot(p,q,'LineWidth',2)\n    axis([0 Scale 0 Scale])\n    \n    j=j+1;\n    M(j)=getframe(gcf);\n    \n    c1=c1+2*Step;\n    c2=c2+2*Step;\n\n    imagenum=imagenum+Step;\n\nend\n    \nmovie2avi(M,F)"("F"=w350, "preSPLINES"=w349, "Scale"=w348, "Step"=w347) -> ()  [unwired: 1 in, 1 out]
        }
      }
    }
  }
  n114 = case shown="True" "Save extra splines\n(at increment)\nto txt file" {
    tunnel: w2 -> [_ w358]
    tunnel: w4 -> [_ w357]
    tunnel: w3 -> [_ w356]
    frame False {
    }
    frame True {
      n115 = Quotient & Remainder(x=w356, y="Increment for\nsaving extra\n splines") -> (floor(x/y)=w352:i32)  [unwired: 1 out]
      n116 = Quotient & Remainder(x=w352, y=2) -> (x-y*floor(x/y)=w351:i32)  [unwired: 1 out]
      n117 = Equal To 0?(x=w351) -> (x = 0?=w355:bool)
      n118 = case shown="True" w355 {
        tunnel: [w364 w366] -> w353
        tunnel: w352 -> [w365 w366]
        frame False {
          n119 = Increment(x=w365) -> (x+1=w364:i32)
        }
        frame True {
        }
      }
      n120 = Initialize Array "Initialize Array \nto store extra splines"(0.0 ("element"), w357, w353) -> (w360:dbl[][])
      n121 = while {
        tunnel: "Increment for\nsaving extra\n splines" -> [w371]
        tunnel: w356 -> [w370]
        shift-right: [w381] -> w361
        shift-left: w360 -> [w379]
        tunnel: w358 -> [w377]
        i -> [w367]
        stop <- w382 stop-if-true
        n122 = Multiply(x=w371, y=2) -> (x*y=w376:i32)
        n123 = Multiply(x=w376, y=w367) -> (x*y=w369:i32)
        n124 = Greater?(x=w369, y=w370) -> (0:w382:bool)
        n125 = Index Array "x data"(array=w377, index (col)=w369) -> (element=w378:dbl[])  [unwired: 1 in]
        n126 = Increment(x=w369) -> (x+1=w380:i32)
        n127 = Multiply(x=w367, y=2) -> (x*y=w373:i32)
        n128 = Increment(x=w373) -> (x+1=w372:i32)
        n129 = Index Array "y data"(array=w377, index (col)=w380) -> (element=w368:dbl[])  [unwired: 1 in]
        n130 = Replace Array Subset "store extra splines"(array=w379, new element #1=w378, index (col) #1=w373, new element #2=w368, index (col) #2=w372) -> (w381:dbl[][])  [unwired: 2 in]
      }
      n131 = call-poly <vilib>:"Write To Spreadsheet File.vi"("2D data"=w361, "file path (dialog if empty)"="File path for extra kinematics splines (dialog if empty)") -> ()  [unwired: 6 in, 1 out]
    }
  }
  n132 = case shown="True" "ON for 2 foil\nsegments" {
    tunnel: w26 -> [w384 w428]
    tunnel: "Number of\ncycles" -> [w388 w427]
    tunnel: w4 -> [_ w426]
    tunnel: w3 -> [_ w425]
    tunnel: "Save splines\nfor snapshot\ngeneration" -> [w389 w424]
    tunnel: w2 -> [_ w423]
    tunnel: w6 -> [w387 _]
    tunnel: w5 -> [w386 _]
    tunnel: w1 -> [w385 _]
    tunnel: "File path for snapshot splines (dialog if empty)" -> [w383 w422]
    frame True {
      n133 = case shown="True" w389 {
        tunnel: w384 -> [_ w399]
        tunnel: w388 -> [_ w397]
        tunnel: w387 -> [_ w393]
        tunnel: w386 -> [_ w392]
        tunnel: w385 -> [_ w391]
        tunnel: w383 -> [_ w390]
        frame False {
        }
        frame True {
          w398 = 24  # Splines per cycle
          n134 = Multiply "Splines\nneeded"(x=w397, y=w398) -> (x*y=w395:i32)
          n135 = Multiply "2 col\nper spline"(x=w395, y=2) -> (x*y=w396:i32)
          n136 = Initialize Array "Initialize Array \nto store snapshots"(0.0 ("element"), w393, w396) -> (w400:dbl[][])
          n137 = while {
            tunnel: w399 -> [w411]
            shift-right: [w420] -> w401
            shift-left: w400 -> [w418]
            tunnel: w391 -> [w416]
            tunnel: w392 -> [w403]
            i -> [w408]
            stop <- w421 stop-if-true
            n138 = Divide(x=w411, y=24.0) -> (x/y=w409:dbl)
            n139 = Multiply(x=w408, y=w409) -> (x*y=w407:dbl)
            n140 = Round To Nearest(number=w407) -> (nearest integer value=w406:dbl)
            n141 = Multiply(x=w406, y=2.0) -> (x*y=w405:dbl)
            n142 = Greater?(x=w405, y=w403) -> (0:w421:bool)
            n143 = Index Array "x data"(array=w416, index (col)=w405) -> (element=w417:dbl[])  [unwired: 1 in]
            n144 = Increment(x=w405) -> (x+1=w419:dbl)
            n145 = Multiply(x=w408, y=2) -> (x*y=w414:i32)
            n146 = Increment(x=w414) -> (x+1=w413:i32)
            n147 = Index Array "y data"(array=w416, index (col)=w419) -> (element=w412:dbl[])  [unwired: 1 in]
            n148 = Replace Array Subset "store\nsnapshots"(array=w418, new element #1=w417, index (col) #1=w414, new element #2=w412, index (col) #2=w413) -> (w420:dbl[][])  [unwired: 2 in]
          }
          n149 = call-poly <vilib>:"Write To Spreadsheet File.vi"("2D data"=w401, "file path (dialog if empty)"=w390) -> ()  [unwired: 6 in, 1 out]
        }
      }
    }
    frame False {
      n150 = case shown="True" w424 {
        tunnel: w428 -> [_ w438]
        tunnel: w427 -> [_ w436]
        tunnel: w426 -> [_ w432]
        tunnel: w425 -> [_ w431]
        tunnel: w423 -> [_ w430]
        tunnel: w422 -> [_ w429]
        frame False {
        }
        frame True {
          w437 = 24  # Splines per cycle
          n151 = Multiply "Splines\nneeded"(x=w436, y=w437) -> (x*y=w434:i32)
          n152 = Multiply "2 col\nper spline"(x=w434, y=2) -> (x*y=w435:i32)
          n153 = Initialize Array "Initialize Array \nto store snapshots"(0.0 ("element"), w432, w435) -> (w439:dbl[][])
          n154 = while {
            tunnel: w438 -> [w450]
            shift-right: [w459] -> w440
            shift-left: w439 -> [w457]
            tunnel: w430 -> [w455]
            tunnel: w431 -> [w442]
            i -> [w447]
            stop <- w460 stop-if-true
            n155 = Divide(x=w450, y=24.0) -> (x/y=w448:dbl)
            n156 = Multiply(x=w447, y=w448) -> (x*y=w446:dbl)
            n157 = Round To Nearest(number=w446) -> (nearest integer value=w445:dbl)
            n158 = Multiply(x=w445, y=2.0) -> (x*y=w444:dbl)
            n159 = Greater?(x=w444, y=w442) -> (0:w460:bool)
            n160 = Index Array "x data"(array=w455, index (col)=w444) -> (element=w456:dbl[])  [unwired: 1 in]
            n161 = Increment(x=w444) -> (x+1=w458:dbl)
            n162 = Multiply(x=w447, y=2) -> (x*y=w453:i32)
            n163 = Increment(x=w453) -> (x+1=w452:i32)
            n164 = Index Array "y data"(array=w455, index (col)=w458) -> (element=w451:dbl[])  [unwired: 1 in]
            n165 = Replace Array Subset "store\nsnapshots"(array=w457, new element #1=w456, index (col) #1=w453, new element #2=w451, index (col) #2=w452) -> (w459:dbl[][])  [unwired: 2 in]
          }
          n166 = call-poly <vilib>:"Write To Spreadsheet File.vi"("2D data"=w440, "file path (dialog if empty)"=w429) -> ()  [unwired: 6 in, 1 out]
        }
      }
    }
  }
  n167 = case shown="True" "ON for 2 foil\nsegments" {
    tunnel: w26 -> [w463 w583]
    tunnel: "Number of\ncycles" -> [w464 w582]
    tunnel: w4 -> [_ w581]
    tunnel: w3 -> [_ w580]
    tunnel: w2 -> [_ w579]
    tunnel: "Save amps of\noscillation\nto txt file" -> [w468 w578]
    tunnel: w1 -> [w467 _]
    tunnel: w6 -> [w466 _]
    tunnel: w5 -> [w465 _]
    tunnel: "Foil chord (m)" -> [w462 w577]
    tunnel: "File path for amplitudes of oscillation (dialog if empty)" -> [w461 w576]
    frame True {
      n168 = case shown="True" w468 {
        tunnel: w463 -> [_ w477]
        tunnel: w464 -> [_ w474]
        tunnel: w466 -> [_ w473]
        tunnel: w465 -> [_ w471]
        tunnel: w467 -> [_ w472]
        tunnel: w462 -> [_ w470]
        tunnel: w461 -> [_ w469]
        frame False {
        }
        frame True {
          n169 = Divide(x=w471, y=2) -> (x/y=w476:dbl)
          n170 = Initialize Array "Initialize Array to\ncalculate amplitudes"(0.0 ("element"), w473, w476) -> (w479:dbl[][])
          n171 = while {
            shift-right: [w504] -> w478
            shift-left: w479 -> [w505]
            tunnel: w472 -> [w502]
            tunnel: w471 -> [w497]
            i -> [w501]
            stop <- w496 stop-if-true
            n172 = Multiply(x=w501, y=2) -> (x*y=w499:i32)
            n173 = Increment(x=w499) -> (x+1=w498:i32)
            n174 = Greater?(x=w498, y=w497) -> (0:w496:bool)
            n175 = Index Array "y data"(array=w502, index (col)=w498) -> (element=w503:dbl[])  [unwired: 1 in]
            n176 = Replace Array Subset "to calculate amps"(array=w505, new element=w503, index (col)=w501) -> (w504:dbl[][])  [unwired: 1 in]
          }
          n177 = Delete From Array "erase header row"(array=w478, index (row)=0) -> (array with subset deleted=w481:dbl[][])  [unwired: 2 in, 1 out]
          n178 = Initialize Array "initialize array\nfor amps"(0.0 ("element"), 1 ("dimension size"), 4 ("dimension size")) -> (w486:dbl[][])
          n179 = for {
            N: w474 -> [_]
            tunnel: w481 -> [w521]
            tunnel: w477 -> [w507]
            shift-right: [w512] -> w485
            shift-left: w486 -> [w513]
            tunnel: w470 -> [w506]
            i -> [w510]
            n180 = Multiply(x=w510, y=w507) -> (x*y=w511:dbl)
            n181 = Initialize Array "Initialize Array\nfor cycle's amps"(0.0 ("element"), 13 ("dimension size"), 4 ("dimension size")) -> (w517:dbl[][])
            n182 = Array Subset "get splines for\ncurrent cycle"(array=w521, index (col)=w511, length (col)=w507) -> (w508:dbl[][])  [unwired: 2 in]
            n183 = Increment(x=w510) -> (x+1=w509:i32)
            n184 = for {
              N: 13 -> [_]
              tunnel: w508 -> [w530]
              shift-right: [w532] -> w516
              shift-left: w517 -> [w533]
              tunnel: w509 -> [w524]
              tunnel: w506 -> [w523]
              i -> [w525]
              n185 = Multiply(x=w525, y=17) -> (x*y=w529:i32)
              n186 = Equal?(x=w525, y=12) -> (x = y?=w526:bool)
              n187 = case shown="False" w526 {
                tunnel: w530 -> [w550 w570]
                tunnel: w529 -> [w549 _]
                tunnel: w525 -> [w547 _]
                tunnel: [w545 w567] -> w528
                tunnel: w523 -> [w541 w564]
                tunnel: w524 -> [w540 w562]
                frame False {
                  n188 = Index Array "choose row (y pos)\nfor given distance\ndown foil"(array=w550, index (row)=w549) -> (element=w551:dbl[])  [unwired: 1 in]
                  n189 = Array Max & Min(array=w551) -> (max value=w536:dbl, min value=w535:dbl)  [unwired: 2 out]
                  n190 = Not Equal To 0?(x=w536) -> (x != 0?=w537:bool)
                  n191 = Equal To 0?(x=w535) -> (x = 0?=w538:bool)
                  n192 = And(x=w537, y=w538) -> (x .and. y?=w539:bool)
                  n193 = case shown="False" w539 {
                    tunnel: [w552 0] -> w534
                    tunnel: w536 -> [w554 _]
                    tunnel: w535 -> [w553 _]
                    frame False {
                      n194 = Subtract(x=w554, y=w553) -> (x-y=w552:dbl)
                    }
                    frame True {
                    }
                  }
                  n195 = Divide(x=w534, y=1000.0) -> (x/y=w542:dbl)
                  n196 = Divide(x=w542, y=w541) -> (x/y=w544:dbl)
                  n197 = Divide(x=w547, y=12) -> (x/y=w548:dbl)
                  n198 = Build Array(w540, w548, w542, w544) -> (w545:dbl[])
                }
                frame True {
                  n199 = Index Array "choose row (y pos)\nfor trailing edge"(array=w570, index (row)=203) -> (element=w571:dbl[])  [unwired: 1 in]
                  n200 = Array Max & Min(array=w571) -> (max value=w558:dbl, min value=w557:dbl)  [unwired: 2 out]
                  n201 = Not Equal To 0?(x=w558) -> (x != 0?=w559:bool)
                  n202 = Equal To 0?(x=w557) -> (x = 0?=w560:bool)
                  n203 = And(x=w559, y=w560) -> (x .and. y?=w561:bool)
                  n204 = case shown="False" w561 {
                    tunnel: [w572 0] -> w556
                    tunnel: w558 -> [w574 _]
                    tunnel: w557 -> [w573 _]
                    frame False {
                      n205 = Subtract(x=w574, y=w573) -> (x-y=w572:dbl)
                    }
                    frame True {
                    }
                  }
                  n206 = Divide(x=w556, y=1000.0) -> (x/y=w565:dbl)
                  n207 = Divide(x=w565, y=w564) -> (x/y=w563:dbl)
                  n208 = Build Array(w562, 1.0 ("element"), w565, w563) -> (w567:dbl[])
                }
              }
              n209 = Replace Array Subset "store amps\nfor cycle"(array=w533, new element=w528, index (row)=w525) -> (w532:dbl[][])  [unwired: 1 in]
            }
            n210 = Multiply(x=13, y=w510) -> (x*y=w515:i32)
            n211 = Insert Into Array "store cycle's amps\nin master list"(array=w513, index (row)=w515, new element=w516) -> (w512:dbl[][])  [unwired: 1 in]
          }
          n212 = Multiply(x=13, y=w474) -> (x*y=w483:i32)
          n213 = Delete From Array "delete empty\nheader row"(array=w485, index (row)=w483) -> (array with subset deleted=w484:dbl[][])  [unwired: 2 in, 1 out]
          n214 = call-poly <vilib>:"Write To Spreadsheet File.vi"("append to file? (new file:F)"=TRUE, "1D data"=string[] ["Cycle number", "Position on foil (L)", "Amplitude of oscillation (m)", "Normalized amplitude (L)"], "file path (dialog if empty)"=w469) -> ("new file path (Not A Path if cancelled)"=w491:path)  [unwired: 5 in]
          n215 = call-poly <vilib>:"Write To Spreadsheet File.vi"("format (%.3f)"="%.5f", "append to file? (new file:F)"=TRUE, "2D data"=w484, "file path (dialog if empty)"=w491) -> ()  [unwired: 4 in, 1 out]
        }
      }
    }
    frame False {
      n216 = case shown="True" w578 {
        tunnel: w583 -> [_ w592]
        tunnel: w582 -> [_ w589]
        tunnel: w581 -> [_ w588]
        tunnel: w580 -> [_ w587]
        tunnel: w579 -> [_ w586]
        tunnel: w577 -> [_ w585]
        tunnel: w576 -> [_ w584]
        frame False {
        }
        frame True {
          n217 = Divide(x=w587, y=2) -> (x/y=w591:dbl)
          n218 = Initialize Array "Initialize Array to\ncalculate amplitudes"(0.0 ("element"), w588, w591) -> (w594:dbl[][])
          n219 = while {
            shift-right: [w619] -> w593
            shift-left: w594 -> [w620]
            tunnel: w586 -> [w617]
            tunnel: w587 -> [w612]
            i -> [w616]
            stop <- w611 stop-if-true
            n220 = Multiply(x=w616, y=2) -> (x*y=w614:i32)
            n221 = Increment(x=w614) -> (x+1=w613:i32)
            n222 = Greater?(x=w613, y=w612) -> (0:w611:bool)
            n223 = Index Array "y data"(array=w617, index (col)=w613) -> (element=w618:dbl[])  [unwired: 1 in]
            n224 = Replace Array Subset "to calculate amps"(array=w620, new element=w618, index (col)=w616) -> (w619:dbl[][])  [unwired: 1 in]
          }
          n225 = Delete From Array "erase header row"(array=w593, index (row)=0) -> (array with subset deleted=w596:dbl[][])  [unwired: 2 in, 1 out]
          n226 = Initialize Array "initialize array\nfor amps"(0.0 ("element"), 1 ("dimension size"), 4 ("dimension size")) -> (w601:dbl[][])
          n227 = for {
            N: w589 -> [_]
            tunnel: w596 -> [w636]
            tunnel: w592 -> [w622]
            shift-right: [w627] -> w600
            shift-left: w601 -> [w628]
            tunnel: w585 -> [w621]
            i -> [w625]
            n228 = Multiply(x=w625, y=w622) -> (x*y=w626:dbl)
            n229 = Initialize Array "Initialize Array\nfor cycle's amps"(0.0 ("element"), 13 ("dimension size"), 4 ("dimension size")) -> (w632:dbl[][])
            n230 = Array Subset "get splines for\ncurrent cycle"(array=w636, index (col)=w626, length (col)=w622) -> (w623:dbl[][])  [unwired: 2 in]
            n231 = Increment(x=w625) -> (x+1=w624:i32)
            n232 = for {
              N: 13 -> [_]
              tunnel: w623 -> [w645]
              shift-right: [w647] -> w631
              shift-left: w632 -> [w648]
              tunnel: w624 -> [w639]
              tunnel: w621 -> [w638]
              i -> [w640]
              n233 = Multiply(x=w640, y=17) -> (x*y=w644:i32)
              n234 = Equal?(x=w640, y=12) -> (x = y?=w641:bool)
              n235 = case shown="False" w641 {
                tunnel: w645 -> [w660 w672]
                tunnel: w644 -> [w659 _]
                tunnel: w640 -> [w657 _]
                tunnel: [w655 w669] -> w643
                tunnel: w638 -> [w650 w666]
                tunnel: w639 -> [w649 w664]
                frame False {
                  n236 = Index Array "choose row (y pos)\nfor given distance\ndown foil"(array=w660, index (row)=w659) -> (element=w661:dbl[])  [unwired: 1 in]
                  n237 = Array Max & Min(array=w661) -> (max value=w662:dbl, min value=w663:dbl)  [unwired: 2 out]
                  n238 = Subtract(x=w662, y=w663) -> (x-y=w653:dbl)
                  n239 = Divide(x=w653, y=1000.0) -> (x/y=w651:dbl)
                  n240 = Divide(x=w651, y=w650) -> (x/y=w654:dbl)
                  n241 = Divide(x=w657, y=12) -> (x/y=w658:dbl)
                  n242 = Build Array(w649, w658, w651, w654) -> (w655:dbl[])
                }
                frame True {
                  n243 = Index Array "choose row (y pos)\nfor trailing edge"(array=w672, index (row)=203) -> (element=w674:dbl[])  [unwired: 1 in]
                  n244 = Array Max & Min(array=w674) -> (max value=w675:dbl, min value=w676:dbl)  [unwired: 2 out]
                  n245 = Subtract(x=w675, y=w676) -> (x-y=w673:dbl)
                  n246 = Divide(x=w673, y=1000.0) -> (x/y=w667:dbl)
                  n247 = Divide(x=w667, y=w666) -> (x/y=w665:dbl)
                  n248 = Build Array(w664, 1.0 ("element"), w667, w665) -> (w669:dbl[])
                }
              }
              n249 = Replace Array Subset "store amps\nfor cycle"(array=w648, new element=w643, index (row)=w640) -> (w647:dbl[][])  [unwired: 1 in]
            }
            n250 = Multiply(x=13, y=w625) -> (x*y=w630:i32)
            n251 = Insert Into Array "store cycle's amps\nin master list"(array=w628, index (row)=w630, new element=w631) -> (w627:dbl[][])  [unwired: 1 in]
          }
          n252 = Multiply(x=13, y=w589) -> (x*y=w598:i32)
          n253 = Delete From Array "delete empty\nheader row"(array=w600, index (row)=w598) -> (array with subset deleted=w599:dbl[][])  [unwired: 2 in, 1 out]
          n254 = call-poly <vilib>:"Write To Spreadsheet File.vi"("append to file? (new file:F)"=TRUE, "1D data"=string[] ["Cycle number", "Position on foil (L)", "Amplitude of oscillation (m)", "Normalized amplitude (L)"], "file path (dialog if empty)"=w584) -> ("new file path (Not A Path if cancelled)"=w606:path)  [unwired: 5 in]
          n255 = call-poly <vilib>:"Write To Spreadsheet File.vi"("format (%.3f)"="%.5f", "append to file? (new file:F)"=TRUE, "2D data"=w599, "file path (dialog if empty)"=w606) -> ()  [unwired: 4 in, 1 out]
        }
      }
    }
  }
